vi "Actor Core.vi"(8 "error in":errorcluster, 11 "Cobra GUI in":refnum<class "Cobra GUI.lvclass">) -> (0 "error out":errorcluster={"status"=TRUE, "code"=1, "source"="Generate User Event in Panel Actor.lvlib:Panel Actor.lvclass:Actor Core.vi:5880001->GUI.lvlib:Cobra GUI.lvclass:Actor Core.vi"}, 3 "Actor out":refnum<class "Actor.lvclass">)   [LabVIEW 2019, in "Cobra GUI.lvlib" / "Cobra GUI.lvclass"]
doc: "New Cobra GUI 21.6.18"
uses:
  Cobra GUI.lvclass
  <vilib>/MGI/Panel Manager/Panel Actor/Panel Actor/Panel Actor.lvclass
  <vilib>/ActorFramework/Stop Msg/Stop Msg.lvclass
  <vilib>/MGI/Panel Manager/Panel/Panel.lvlib
  TTV Test/TTV Test/TTV Test.lvclass
  GUI 1.0/Controls/System Graphs.ctl
  GUI 1.0/GUI.lvlib
  GUI 1.0/Controls/Gauge Graphs/Compression Ratio.ctl
  GUI 1.0/Controls/Gauge Graphs/Subcooling.ctl
  GUI 1.0/Controls/Gauge Graphs/Superheat.ctl
  GUI 1.0/Controls/Gauge Graphs/Current.ctl
  GUI 1.0/Controls/Dial Gauges.ctl
  GUI Messages/Save Config Msg/Save Config Msg.lvclass
  Custom Controls/login.ctl
  <vilib>/Utility/miscctls.llb/LVPositionTypeDef.ctl
  Network Stream Messages/Open Connection Msg/Open Connection Msg.lvclass
  Network Stream/Network Stream Messages/Read Dataset Msg/Read Dataset Msg.lvclass
  Network Stream/Network Stream Messages/Close Connection Msg/Close Connection Msg.lvclass
  GUI 1.0/Controls/NS New Data.ctl
  GUI 1.0/Controls/WebDAV states.ctl
  GUI Messages/Update Msg/Update Msg.lvclass
  <vilib>/regexp/Match Regular Expression.xnode
  GUI Messages/Get IP Address Msg/Get IP Address Msg.lvclass
  <vilib>/MGI/Panel Manager/Panel/Panel/Subpanel/Subpanel.vi
  <vilib>/MGI/Panel Manager/Panel/Panel/Subpanel/Subpanel.lvclass
  C:/Program Files (x86)/National Instruments/LabVIEW 2019/vi.lib/MGI/Panel Manager/Panel Actor/Panel Actor/Panel Actor.lvclass
  C:/Program Files (x86)/National Instruments/LabVIEW 2019/vi.lib/MGI/Monitored Actor/Monitored Actor/Monitored Actor/Monitored Actor.lvclass
  C:/Program Files (x86)/National Instruments/LabVIEW 2019/vi.lib/ActorFramework/Actor/Actor.lvclass
  C:/Program Files (x86)/National Instruments/LabVIEW 2019/vi.lib/MGI/Panel Manager/Panel/Panel/Panel.lvclass
  <vilib>/ActorFramework/Actor/Actor.lvclass
  GUI 1.0/Controls/Module Key Values.ctl
  Private Controls/Module Command.ctl
  GUI 1.0/Controls/Main Waveform.ctl
  Custom Controls/Head State and Wait for the safe temp.ctl
  <vilib>/ActorFramework/Message Enqueuer/Message Enqueuer.lvclass
  <vilib>/ActorFramework/Message Priority Queue/Message Priority Queue.lvclass
  <vilib>/MGI/Panel Manager/Panel/Panel/Panel.lvclass
  <vilib>/MGI/Panel Manager/Panel/Panel Helper/Panel Helper.lvclass
  <vilib>/MGI/Panel Manager/Panel/Deferer/Deferer.lvclass
  <vilib>/MGI/Panel Manager/Panel/Panel Control Counter/Panel Control Counter.lvclass
  GUI 1.0/Controls/Module Graphs.ctl
panel:
  out "IP Address":string
  out "Connected System":string="Connected"
  out "System Info":string="Connected"
  in  "Tab Control":T1(tab)=enum."Debug"
  in  "M1 Power Drive":bool
  in  "M2 Power Drive":bool
  out "M2 Safe Temp and Head State":T2
  out "M1 Safe Temp and Head State":T2
  in  "Power On-Off":bool
  out "M2 Main Waveform":T3=[{"t0"=timestamp(3697564714.4984064 s since 1904-01-01), "dt"=1.0, "Y"=array[1697 elements]}, {"t0"=timestamp(3697564714.4984064 s since 1904-01-01), "dt"=1.0, "Y"=array[1697 elements]}, {"t0"=timestamp(3697564714.4984064 s since 1904-01-01), "dt"=1.0, "Y"=array[1697 elements]}, {"t0"=timestamp(3697564714.4984064 s since 1904-01-01), "dt"=1.0, "Y"=array[1697 elements]}]
  out "M1 Main Waveform":T3=[{"t0"=timestamp(3697564714.4984064 s since 1904-01-01), "dt"=1.0, "Y"=array[1697 elements]}, {"t0"=timestamp(3697564714.4984064 s since 1904-01-01), "dt"=1.0, "Y"=array[1697 elements]}, {"t0"=timestamp(3697564714.4984064 s since 1904-01-01), "dt"=1.0, "Y"=array[1697 elements]}, {"t0"=timestamp(3697564714.4984064 s since 1904-01-01), "dt"=1.0, "Y"=array[1697 elements]}]
  in  "M1 Commands":T4={"Set Temp"=273.15, "Read Temp"=273.15, "Package"=0, "Bin String"="", "M1 Enable"=TRUE, "TSD"=TRUE} caption="Module Commands" {"Package" items=["Ring", "Item 1", "Item 2", "Item 3"]; "Set Temp" format="%#4.1f"}
  in  "M2 Commands":T4={"Set Temp"=273.15, "Read Temp"=273.15, "Package"=0, "Bin String"="", "M1 Enable"=TRUE, "TSD"=TRUE} caption="Module Commands" {"Package" items=["Ring", "Item 1", "Item 2", "Item 3"]; "Set Temp" format="%#4.1f"}
  out "M1 Humidity":cluster{"M1 RH":dbl, "RH Threshold":dbl}(graph)={"M1 RH"=10.0, "RH Threshold"=33.76176771953824}
  out "Thermal Info":T5={"M1 Thermal State"=enum."Steady State", "M2 Thermal State"=enum."Ramp Up", "High Side RPM"=0.0, "Low Side RPM"=0.0}
  out "System Graphs":T6={"Ambient Temp"=77.534379824996, "Suction Temp"=77.78750485181808, "Condensor Temp"=77.29531729966402, "Discharge Temp"=78.09687988460064, "Bypass Steps"=72.0}
  out "Gauges":T7={"Condensing Pressure(psi)"=165.57116807812622, "Compression Ratio"=1.0119646390563775, "Subcool"=-0.3368072880168427, "Superheat"=1.4200558413526494, "Current(A)"=0.2333286882987343, "Suction Pressure(psi)"=163.4397897916897} {"Suction Pressure(psi)" scale=0.0..100.0; "Current(A)" scale=5.0..15.0 scale format="%_1f"; "Superheat" scale=0.0..100.0; "Subcool" scale=-10.0..20.0 scale format="%#4.1f"; "Compression Ratio" scale=0.0..30.0 scale format="%#.0f"; "Condensing Pressure(psi)" scale=150.0..375.0}
  in  "Graph Tab CTL":enum32{"Head #1", "Head #2"}(tab)
  out "M1 Graphs":T12={"Case Temp"=24.9375, "Evap Temp"=24.8046875, "Heater Power (%)"=0.0, "EEV Steps"=0.0, "M1 AC Load(W)"=10.492394664499656} caption="Head #1"
  out "M2 Graphs":T12 caption="Head #2"
  out "Errors":string[](array[string])=["Warning: Air not plugged in  (21 06 08 14 08)"]
  out "Event log":T13(array[cluster])=[{"Name"="Bypass Inintialized", "Time Stamp"=timestamp(3706031317.901618 s since 1904-01-01), "Code"="", "Source"="", "Value"=22160.0, "Boolean"=FALSE, "String"="Complete", "Error"=FALSE, "Warning"=FALSE, " Fault"=FALSE}, {"Name"="Timeserver not found", "Time Stamp"=timestamp(3706031309.741007 s since 1904-01-01), "Code"="", "Source"="SOM Time", "Value"=0.0, "Boolean"=FALSE, "String"="", "Error"=FALSE, "Warning"=FALSE, " Fault"=FALSE}, {"Name"="Bypass Target Change", "Time Stamp"=timestamp(3706031309.711301 s since 1904-01-01), "Code"="", "Source"="Bypass:Get Target", "Value"=110.0, "Boolean"=FALSE, "String"="", "Error"=FALSE, "Warning"=TRUE, " Fault"=FALSE}, {"Name"="Mains Frequency", "Time Stamp"=timestamp(3706031309.198055 s since 1904-01-01), "Code"="", "Source"="Init System Module", "Value"=59.9940002520096, "Boolean"=FALSE, "String"="", "Error"=FALSE, "Warning"=FALSE, " Fault"=FALSE}, {"Name"="PID Bypassed", "Time Stamp"=timestamp(3706031307.313306 s since 1904-01-01), "Code"="", "Source"="APP:Set/Send PID Bypass", "Value"=0.0, "Boolean"=FALSE, "String"="", "Error"=FALSE, "Warning"=FALSE, " Fault"=FALSE}, {"Name"="Thermal Status Change", "Time Stamp"=timestamp(3706031307.007236 s since 1904-01-01), "Code"="", "Source"="APP:Thermal Status", "Value"=0.0, "Boolean"=FALSE, "String"="", "Error"=FALSE, "Warning"=FALSE, " Fault"=FALSE}, {"Name"="Feedback Change", "Time Stamp"=timestamp(3706031306.793005 s since 1904-01-01), "Code"="", "Source"="APP:Get Feedback", "Value"=1.0, "Boolean"=FALSE, "String"="Case", "Error"=FALSE, "Warning"=FALSE, " Fault"=FALSE}, {"Name"="M1 Setpoint Change", "Time Stamp"=timestamp(3706031306.436291 s since 1904-01-01), "Code"="", "Source"="APP:Send Set Temp", "Value"=25.0, "Boolean"=FALSE, "String"="", "Error"=FALSE, "Warning"=TRUE, " Fault"=FALSE}, {"Name"="M1 Dynamic Set Point", "Time Stamp"=timestamp(3706031306.386277 s since 1904-01-01), "Code"="", "Source"="APP:Get Dynamic Set Temp", "Value"=25.0, "Boolean"=FALSE, "String"="", "Error"=FALSE, "Warning"=FALSE, " Fault"=FALSE}, {"Name"="M1 EEV Check Position", "Time Stamp"=timestamp(3706031306.325976 s since 1904-01-01), "Code"="", "Source"="", "Value"=0.0, "Boolean"=TRUE, "String"="Complete", "Error"=FALSE, "Warning"=FALSE, " Fault"=FALSE}, {"Name"="I2C TSD Freeze Timeout", "Time Stamp"=timestamp(3706031300.268274 s since 1904-01-01), "Code"="", "Source"="", "Value"=0.0, "Boolean"=FALSE, "String"="", "Error"=TRUE, "Warning"=FALSE, " Fault"=FALSE}, {"Name"="New Extra Settings Loaded", "Time Stamp"=timestamp(3706031298.435066 s since 1904-01-01), "Code"="", "Source"="", "Value"=0.0, "Boolean"=FALSE, "String"="", "Error"=FALSE, "Warning"=FALSE, " Fault"=FALSE}, {"Name"="Read Compressor Minutes", "Time Stamp"=timestamp(3706031298.210019 s since 1904-01-01), "Code"="", "Source"="", "Value"=0.0, "Boolean"=TRUE, "String"="PASS", "Error"=FALSE, "Warning"=FALSE, " Fault"=FALSE}, {"Name"="M1 EEV Check Position", "Time Stamp"=timestamp(3706031296.21211 s since 1904-01-01), "Code"="", "Source"="EEV:Check Position", "Value"=0.0, "Boolean"=FALSE, "String"="", "Error"=FALSE, "Warning"=FALSE, " Fault"=FALSE}, {"Name"="EEV PID Output", "Time Stamp"=timestamp(3706031296.161288 s since 1904-01-01), "Code"="", "Source"="APP:Send EEV PID Out", "Value"=0.0, "Boolean"=FALSE, "String"="Value Change", "Error"=FALSE, "Warning"=FALSE, " Fault"=FALSE}, {"Name"="", "Time Stamp"=timestamp(3706031296.053791 s since 1904-01-01), "Code"="", "Source"="EEV:Set Position", "Value"=0.0, "Boolean"=FALSE, "String"="", "Error"=FALSE, "Warning"=FALSE, " Fault"=FALSE}, {"Name"="", "Time Stamp"=timestamp(3706031296.000374 s since 1904-01-01), "Code"="", "Source"="EEV:Config", "Value"=0.0, "Boolean"=FALSE, "String"="", "Error"=FALSE, "Warning"=FALSE, " Fault"=FALSE}, {"Name"="M1 EEV Check Position", "Time Stamp"=timestamp(3706031294.611185 s since 1904-01-01), "Code"="", "Source"="", "Value"=2000.0, "Boolean"=TRUE, "String"="Complete", "Error"=FALSE, "Warning"=FALSE, " Fault"=FALSE}, {"Name"="M1 EEV Check Position", "Time Stamp"=timestamp(3706031294.000098 s since 1904-01-01), "Code"="", "Source"="EEV:Check Position", "Value"=0.0, "Boolean"=FALSE, "String"="", "Error"=FALSE, "Warning"=FALSE, " Fault"=FALSE}, {"Name"="EEV PID Output", "Time Stamp"=timestamp(3706031293.949764 s since 1904-01-01), "Code"="", "Source"="APP:Send EEV PID Out", "Value"=2000.0, "Boolean"=FALSE, "String"="Value Change", "Error"=FALSE, "Warning"=FALSE, " Fault"=FALSE}, {"Name"="", "Time Stamp"=timestamp(3706031293.848812 s since 1904-01-01), "Code"="", "Source"="EEV:Set Position", "Value"=0.0, "Boolean"=TRUE, "String"="", "Error"=FALSE, "Warning"=FALSE, " Fault"=FALSE}, {"Name"="EEV:Set V", "Time Stamp"=timestamp(3706031293.798386 s since 1904-01-01), "Code"="", "Source"="", "Value"=0.0, "Boolean"=FALSE, "String"="", "Error"=FALSE, "Warning"=FALSE, " Fault"=FALSE}, {"Name"="", "Time Stamp"=timestamp(3706031293.748195 s since 1904-01-01), "Code"="", "Source"="EEV:Config", "Value"=0.0, "Boolean"=FALSE, "String"="", "Error"=FALSE, "Warning"=FALSE, " Fault"=FALSE}, {"Name"="Config Loaded", "Time Stamp"=timestamp(3706031293.397414 s since 1904-01-01), "Code"="", "Source"="Config Read Initialize", "Value"=107.0, "Boolean"=FALSE, "String"="", "Error"=FALSE, "Warning"=FALSE, " Fault"=FALSE}, {"Name"="Config Read", "Time Stamp"=timestamp(3706031293.37065 s since 1904-01-01), "Code"="Found", "Source"="EEV PID", "Value"=25.0, "Boolean"=FALSE, "String"="", "Error"=FALSE, "Warning"=FALSE, " Fault"=FALSE}, {"Name"="Config Read", "Time Stamp"=timestamp(3706031293.359371 s since 1904-01-01), "Code"="Found", "Source"="Set Point Range", "Value"=-50.0, "Boolean"=FALSE, "String"="", "Error"=FALSE, "Warning"=FALSE, " Fault"=FALSE}, {"Name"="Config Value Read", "Time Stamp"=timestamp(3706031293.335439 s since 1904-01-01), "Code"="", "Source"="", "Value"=0.0, "Boolean"=TRUE, "String"="Cascade", "Error"=FALSE, "Warning"=FALSE, " Fault"=FALSE}, {"Name"="Config Value Read", "Time Stamp"=timestamp(3706031293.315639 s since 1904-01-01), "Code"="", "Source"="", "Value"=0.0, "Boolean"=TRUE, "String"="Sensors", "Error"=FALSE, "Warning"=FALSE, " Fault"=FALSE}, {"Name"="Read Saved State", "Time Stamp"=timestamp(3706031293.26891 s since 1904-01-01), "Code"="", "Source"="", "Value"=0.0, "Boolean"=FALSE, "String"="", "Error"=FALSE, "Warning"=FALSE, " Fault"=FALSE}, {"Name"="EMO Switch Detected", "Time Stamp"=timestamp(3706031293.21723 s since 1904-01-01), "Code"="", "Source"="", "Value"=0.0, "Boolean"=TRUE, "String"="", "Error"=FALSE, "Warning"=FALSE, " Fault"=FALSE}, {"Name"="Read Saved State", "Time Stamp"=timestamp(3706031293.183574 s since 1904-01-01), "Code"="", "Source"="", "Value"=0.0, "Boolean"=FALSE, "String"="", "Error"=FALSE, "Warning"=FALSE, " Fault"=FALSE}, {"Name"="FPGA Load Complete", "Time Stamp"=timestamp(3706031293.139812 s since 1904-01-01), "Code"="", "Source"="Init FPGA IO.vi", "Value"=0.0, "Boolean"=FALSE, "String"="", "Error"=FALSE, "Warning"=FALSE, " Fault"=FALSE}, {"Name"="Pressure Test", "Time Stamp"=timestamp(3706031291.136962 s since 1904-01-01), "Code"="", "Source"="Init FPGA IO 2.0.vi", "Value"=0.00022888532845044633, "Boolean"=FALSE, "String"="FAIL", "Error"=FALSE, "Warning"=TRUE, " Fault"=FALSE}, {"Name"="Stop LCD", "Time Stamp"=timestamp(3706031285.92111 s since 1904-01-01), "Code"="", "Source"="Init FPGA IO.vi", "Value"=11.0, "Boolean"=FALSE, "String"="", "Error"=FALSE, "Warning"=FALSE, " Fault"=FALSE}, {"Name"="wait", "Time Stamp"=timestamp(3706031284.919174 s since 1904-01-01), "Code"="", "Source"="Init FPGA IO.vi", "Value"=10.0, "Boolean"=FALSE, "String"="", "Error"=FALSE, "Warning"=FALSE, " Fault"=FALSE}, {"Name"="IP Address", "Time Stamp"=timestamp(3706031283.915648 s since 1904-01-01), "Code"="", "Source"="Init FPGA IO.vi", "Value"=12.0, "Boolean"=FALSE, "String"="þQ", "Error"=FALSE, "Warning"=FALSE, " Fault"=FALSE}, {"Name"="wait", "Time Stamp"=timestamp(3706031283.836404 s since 1904-01-01), "Code"="", "Source"="Init FPGA IO.vi", "Value"=10.0, "Boolean"=FALSE, "String"="", "Error"=FALSE, "Warning"=FALSE, " Fault"=FALSE}, {"Name"="Rev Display", "Time Stamp"=timestamp(3706031282.833974 s since 1904-01-01), "Code"="", "Source"="Init FPGA IO.vi", "Value"=9.0, "Boolean"=FALSE, "String"="Ver: CC 21.6.1.0", "Error"=FALSE, "Warning"=FALSE, " Fault"=FALSE}, {"Name"="wait", "Time Stamp"=timestamp(3706031282.765893 s since 1904-01-01), "Code"="", "Source"="Init FPGA IO.vi", "Value"=10.0, "Boolean"=FALSE, "String"="", "Error"=FALSE, "Warning"=FALSE, " Fault"=FALSE}, {"Name"="Chroma Display", "Time Stamp"=timestamp(3706031281.763213 s since 1904-01-01), "Code"="", "Source"="Init FPGA IO.vi", "Value"=8.0, "Boolean"=FALSE, "String"="Chroma ATE", "Error"=FALSE, "Warning"=FALSE, " Fault"=FALSE}, {"Name"="wait", "Time Stamp"=timestamp(3706031281.696552 s since 1904-01-01), "Code"="", "Source"="Init FPGA IO.vi", "Value"=10.0, "Boolean"=FALSE, "String"="", "Error"=FALSE, "Warning"=FALSE, " Fault"=FALSE}, {"Name"="Clear LCD Text", "Time Stamp"=timestamp(3706031280.693969 s since 1904-01-01), "Code"="", "Source"="Init FPGA IO.vi", "Value"=0.0, "Boolean"=FALSE, "String"="", "Error"=FALSE, "Warning"=FALSE, " Fault"=FALSE}, {"Name"="BootLoad", "Time Stamp"=timestamp(3706031279.648552 s since 1904-01-01), "Code"="", "Source"="Init FPGA IO.vi", "Value"=0.0, "Boolean"=FALSE, "String"="", "Error"=FALSE, "Warning"=FALSE, " Fault"=FALSE}, {"Name"="Extra Settings Loaded", "Time Stamp"=timestamp(3706031277.495041 s since 1904-01-01), "Code"="", "Source"="", "Value"=0.0, "Boolean"=FALSE, "String"="", "Error"=FALSE, "Warning"=FALSE, " Fault"=FALSE}, {"Name"="Warmup ", "Time Stamp"=timestamp(3706031277.461598 s since 1904-01-01), "Code"="", "Source"="Extra Settings", "Value"=0.0, "Boolean"=FALSE, "String"="", "Error"=FALSE, "Warning"=TRUE, " Fault"=FALSE}, {"Name"="Flow Curve", "Time Stamp"=timestamp(3706031277.436586 s since 1904-01-01), "Code"="", "Source"="Extra Settings", "Value"=0.0, "Boolean"=FALSE, "String"="", "Error"=FALSE, "Warning"=TRUE, " Fault"=FALSE}, {"Name"="Relative Humidity", "Time Stamp"=timestamp(3706031277.408702 s since 1904-01-01), "Code"="", "Source"="Extra Settings", "Value"=0.0, "Boolean"=TRUE, "String"="", "Error"=FALSE, "Warning"=FALSE, " Fault"=FALSE}, {"Name"="Warnings/Faults 1", "Time Stamp"=timestamp(3706031277.370367 s since 1904-01-01), "Code"="", "Source"="Extra Settings 3", "Value"=0.0, "Boolean"=TRUE, "String"="", "Error"=FALSE, "Warning"=FALSE, " Fault"=FALSE}, {"Name"="SuperHeat Settings", "Time Stamp"=timestamp(3706031277.356517 s since 1904-01-01), "Code"="", "Source"="Extra Settings 3", "Value"=0.0, "Boolean"=TRUE, "String"="", "Error"=FALSE, "Warning"=FALSE, " Fault"=FALSE}, {"Name"="Config Loaded", "Time Stamp"=timestamp(3706031277.313113 s since 1904-01-01), "Code"="", "Source"="Config Read Initialize", "Value"=74.0, "Boolean"=FALSE, "String"="", "Error"=FALSE, "Warning"=FALSE, " Fault"=FALSE}, {"Name"="Config Read", "Time Stamp"=timestamp(3706031277.287857 s since 1904-01-01), "Code"="Found", "Source"="M2 Heater PID", "Value"=0.0, "Boolean"=FALSE, "String"="", "Error"=FALSE, "Warning"=FALSE, " Fault"=FALSE}, {"Name"="Config Value Read", "Time Stamp"=timestamp(3706031277.269987 s since 1904-01-01), "Code"="", "Source"="", "Value"=0.0, "Boolean"=TRUE, "String"="Handler", "Error"=FALSE, "Warning"=FALSE, " Fault"=FALSE}] {"Value" format="%4.1f"; "Time Stamp" format="%<%x %.3X>T"}
  in  "Reboot RT":bool caption="Reboot"
  in  "Login":T14
  in  "Config Data":bool
  in  "Datalog":bool
  out "TCP Connections":T15(array[cluster])=[{"port "=1300, "remote address"="", "Connection timeout ms"=100, "Waiting for connection"=TRUE, "Waiting for Command"=FALSE, "timeout ms"=5000}, {"port "=1100, "remote address"="", "Connection timeout ms"=100, "Waiting for connection"=TRUE, "Waiting for Command"=FALSE, "timeout ms"=-1}, {"port "=1000, "remote address"="", "Connection timeout ms"=100, "Waiting for connection"=TRUE, "Waiting for Command"=FALSE, "timeout ms"=60000}, {"port "=1001, "remote address"="", "Connection timeout ms"=100, "Waiting for connection"=TRUE, "Waiting for Command"=FALSE, "timeout ms"=60000}, {"port "=2100, "remote address"="", "Connection timeout ms"=100, "Waiting for connection"=FALSE, "Waiting for Command"=FALSE, "timeout ms"=-1}, {"port "=2001, "remote address"="", "Connection timeout ms"=100, "Waiting for connection"=FALSE, "Waiting for Command"=FALSE, "timeout ms"=60000}, {"port "=2000, "remote address"="", "Connection timeout ms"=100, "Waiting for connection"=FALSE, "Waiting for Command"=FALSE, "timeout ms"=5000}]
  out "TCP commands":string[](array[string])
  in  "Cascade Compressor controls":T16 {"Manual Low Stage frequency" min=40.0 max=150.0 step=1.0; "Manual High stage frequency" min=50.0 max=150.0 step=1.0}
  in  "Manual Controls":T17
  in  "Tuning":T18={"Login TO"=10, "Fixed Y-Range"=4.0, "Average Graph"=FALSE, "Temp Unit"=FALSE, "Data Rx Timestamp"=timestamp(3700634217.978288 s since 1904-01-01), "Y-scale"=FALSE} {"Login TO" min=-1 max=1000}
  out "M2 Cluster":T19={"M2 Heater %"=0.0, "M2 Actuated"=FALSE, "M2 Error"=FALSE, "M2 Thermal Status"=enum."Steady State", "M2 Head State"=enum."Disabled", "M2 Buffer"=0.9999999999999998, "M2 Valve Output"=0.0} {"M2 Valve Output" scale=0.0..100.0; "M2 Buffer" scale=-4.0..4.0; "M2 Heater %" format="%3.0f"}
  out "M1 Cluster":T20={"M1 Heater %"=0.0, "M1 Actuated"=FALSE, "M1 Error"=FALSE, "M1 Thermal Status"=enum."Steady State", "M1 Head State"=enum."Disabled", "M1 Buffer"=0.9999999999999998, "M1 Valve Output"=0.0} {"M1 Valve Output" scale=0.0..100.0; "M1 Buffer" scale=-4.0..4.0; "M1 Heater %" format="%3.0f"}
  out "System Cluster":T21={"Serial Number"="204300076", "Compressor Hours"=59.65, "SOM Storage(MB)"=243.036, "Memory Available"=353.72, "CPU Usage"=40.953570959266244, "Software Version"="SW Version:CC 21.4.8.1", "SD card free space"=31.886, "Comp Temp"=78.09687988460064, "Sleep Timer"=-1.0, "Sleep"=TRUE, "Boot Up Time"=timestamp(3700144843.654765 s since 1904-01-01)} {"Comp Temp" format="%#.1f"; "SD card free space" format="%#4.1f"; "CPU Usage" format="%#.1f"; "Memory Available" format="%#4.1f"; "SOM Storage(MB)" format="%4.1f"; "Compressor Hours" format="%#.1f"}
  out "RT Status:":string="Running"
  out "Compressor:":string="Running"
  out "M1 State":T22={"Set Temp"=20.0, "Read Temp"=0.0, "Package"="", "Force"=0.0, "Feedback"=1} caption="M1 Status" {"Feedback" items=["Evap Temp", "Case Temp", "Intec Temp", "TSD  Temp", "Autotune", "Extra"]; "Force" format="%4.1f"; "Read Temp" format="%4.1f"; "Set Temp" format="%4.0f"}
  out "M2 State":T22={"Set Temp"=20.0, "Read Temp"=0.0, "Package"="", "Force"=0.0, "Feedback"=1} caption="M2 Status" {"Feedback" items=["Evap Temp", "Case Temp", "Intec Temp", "TSD  Temp", "Autotune", "Extra"]; "Force" format="%4.1f"; "Read Temp" format="%4.1f"; "Set Temp" format="%4.0f"}
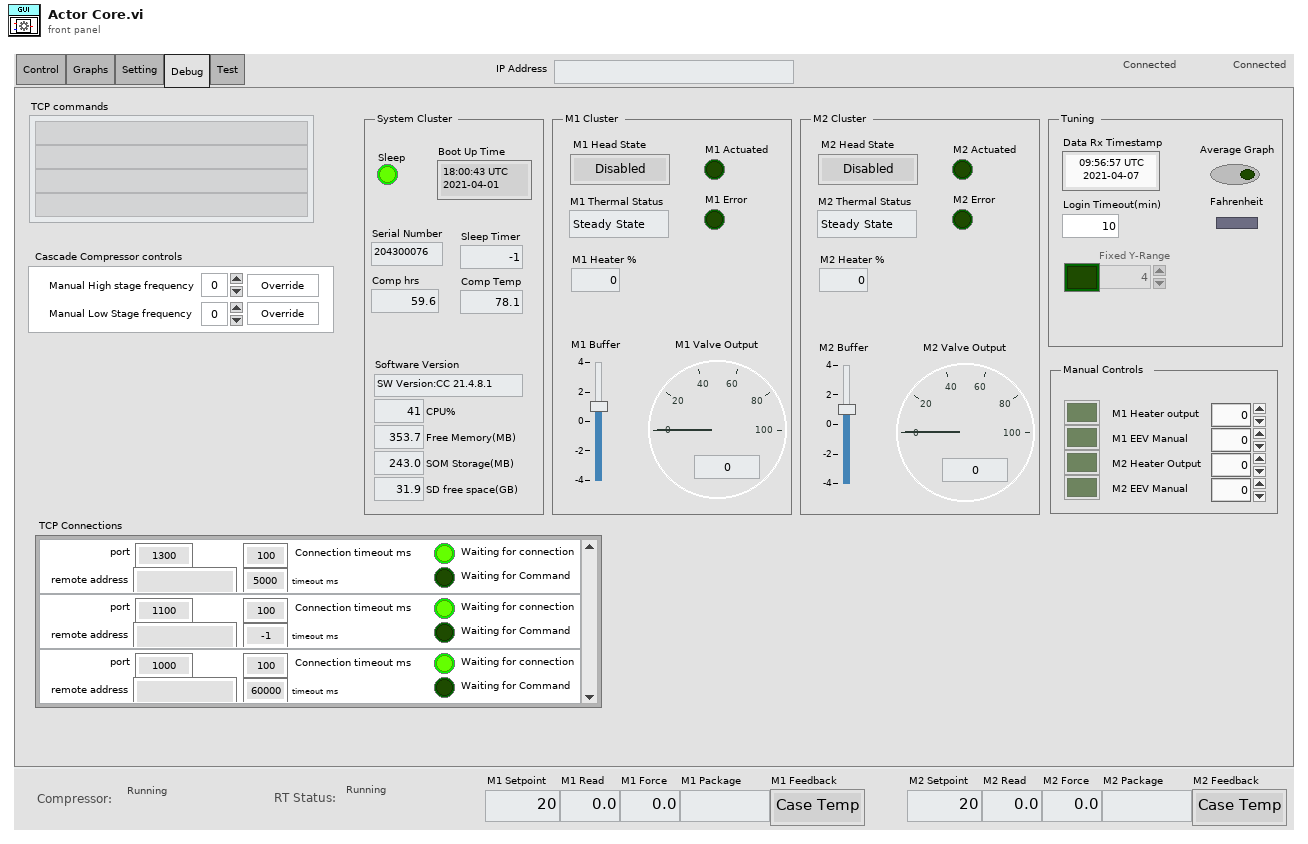
[diagram p1: front panel]
types:
  T1 = enum32{"Control", "Graphs", "Setting", "Debug", "Test"}
  T2 = typedef "GUI.lvlib/Head State and Wait for the safe temp.ctl" = bool
  T3 = typedef "GUI.lvlib/Main Waveform.ctl" = waveform(dbl)[]
  T4 = typedef "LabGUI.lvlib/Module Command.ctl" = cluster{"Set Temp":dbl[unit], "Read Temp":dbl[unit], "Package":u16, "Bin String":string, "M1 Enable":bool, "TSD":bool}
  T5 = cluster{"M1 Thermal State":enum16{"Ramp Up", "Ramp Down", "Steady State", "Ebb and Flow", "Up", "Under Load", "Cryo Mode"}, "M2 Thermal State":enum16{"Ramp Up", "Ramp Down", "Steady State", "Ebb and Flow", "Up", "Under Load", "Cryo Mode", "Shuttle Mode"}, "High Side RPM":dbl, "Low Side RPM":dbl}
  T6 = typedef "GUI.lvlib/System Graphs.ctl" = cluster{"Ambient Temp":dbl, "Suction Temp":dbl, "Condensor Temp":dbl, "Discharge Temp":dbl, "Bypass Steps":dbl}
  T7 = typedef "GUI.lvlib/Dial Gauges.ctl" = cluster{"Condensing Pressure(psi)":dbl, "Compression Ratio":T8, "Subcool":T9, "Superheat":T10, "Current(A)":T11, "Suction Pressure(psi)":dbl}
  T8 = typedef "GUI.lvlib/Compression Ratio.ctl" = dbl
  T9 = typedef "GUI.lvlib/Subcooling.ctl" = dbl
  T10 = typedef "GUI.lvlib/Superheat.ctl" = dbl
  T11 = typedef "GUI.lvlib/Current.ctl" = dbl
  T12 = typedef "GUI.lvlib/Module Graphs.ctl" = cluster{"Case Temp":dbl, "Evap Temp":dbl, "Heater Power (%)":dbl, "EEV Steps":dbl, "M1 AC Load(W)":dbl}
  T13 = cluster{"Name":string, "Time Stamp":timestamp, "Code":string, "Source":string, "Value":dbl, "Boolean":bool, "String":string, "Error":bool, "Warning":bool, " Fault":bool}[]
  T14 = typedef "GUI.lvlib/login.ctl" = bool
  T15 = cluster{"port ":u16, "remote address":string, "Connection timeout ms":i32, "Waiting for connection":bool, "Waiting for Command":bool, "timeout ms":i32}[]
  T16 = cluster{"High Stage manual speed control":bool, "Manual High stage frequency":dbl, "Low Stage manual speed control":bool, "Manual Low Stage frequency":dbl}
  T17 = cluster{"Manual Bypass Mode":bool[], "M1 Heater output":dbl, "M1 EEV Manual":u16, "M2 Heater Output":dbl, "M2 EEV Manual":u16}
  T18 = cluster{"Login TO":i32, "Fixed Y-Range":dbl, "Average Graph":bool, "Temp Unit":bool, "Data Rx Timestamp":timestamp, "Y-scale":bool}
  T19 = cluster{"M2 Heater %":dbl, "M2 Actuated":bool, "M2 Error":bool, "M2 Thermal Status":enum16{"Ramp Up", "Ramp Down", "Steady State", "Ebb and Flow", "Up", "Under Load", "Cryo Mode"}, "M2 Head State":enum16{"Disabled", "Run", "Error"}, "M2 Buffer":dbl, "M2 Valve Output":dbl}
  T20 = cluster{"M1 Heater %":dbl, "M1 Actuated":bool, "M1 Error":bool, "M1 Thermal Status":enum16{"Ramp Up", "Ramp Down", "Steady State", "Ebb and Flow", "Up", "Under Load", "Cryo Mode"}, "M1 Head State":enum16{"Disabled", "Run", "Error"}, "M1 Buffer":dbl, "M1 Valve Output":dbl}
  T21 = cluster{"Serial Number":string, "Compressor Hours":dbl, "SOM Storage(MB)":dbl, "Memory Available":dbl, "CPU Usage":dbl, "Software Version":string, "SD card free space":dbl, "Comp Temp":dbl, "Sleep Timer":dbl, "Sleep":bool, "Boot Up Time":timestamp}
  T22 = typedef "GUI.lvlib/Module Key Values.ctl" = cluster{"Set Temp":dbl, "Read Temp":dbl, "Package":string, "Force":dbl, "Feedback":u8}
  T23 = enum32{"Invalid", "Standard", "Closed", "Hidden", "Minimized", "Maximized"}
  T24 = cluster{"Event Registration Refnum":refnum<event-registration>, "Pnl Actor":refnum<event-registration>}
  T25 = enum32{"Page Enabled", "Page Disabled", "Page Disabled & Grayed"}
  T26 = typedef "LVPositionTypeDef.ctl" = cluster{"Left":i32, "Top":i32}
  T27 = typedef "GUI.lvlib/NS New Data.ctl" = enum16{"M1 Set Point", "M1 Power Drive", "M1 Feedback", "M1 Package", "M1 Enable", "M2 Set Point", "M2 Power Drive", "M2 Feedback", "M2 Package", "M2 Enable", "System Power", "Config Data", "Stop RT"}
  T28 = enum8{"Enabled", "Disabled", "Disabled and Grayed Out"}
  T29 = enum16{"Supervisor", "Engineer", "Operator", "Guest"}
  T30 = typedef "GUI.lvlib/WebDAV states.ctl" = enum16{"Open Sess", "Refresh Dir", "Create Dir", "Upload", "Download", "Delete", "Close Sess"}
  T31 = cluster{"Set Temp":dbl, "Power Drive":bool, "Feedback":u8, "Package":u16, "Enable":bool}
  T32 = typedef "GUI.lvlib/Network Data Down_set back.ctl" = cluster{"M1 Commands":cluster{"Set Temp":dbl, "Power Drive":bool, "Feedback":u8, "Package":u16, "Enable":bool}, "M2 Commands":cluster{"Set Temp":dbl, "Power Drive":bool, "Feedback":u8, "Package ":u16, "Enable":bool}, "Config Data":cluster{"Packages":cluster{"DUT Force lbf":cluster{" 0":u32, " 1":u32, " 2":u32, "3":u32, "4":u32, "5":u32, " 6":u32, "7":u32, "8":u32, "9":u32}, "DUT Names":cluster{"0":string, "1":string, "2":string, "3":string, "4":string, "5":string, "6":string, "7":string, "8":string, "9":string}}, "Heater PID":cluster{"P":dbl, "I":dbl, "D":dbl}, "Piston Settings":cluster{"Forces Slope":dbl, "Forces Intercept":dbl, "Transition Force":dbl, "Up Force":dbl, "Diameter (mm)":dbl, "Delay (ms)":dbl, "Pressure Ramp Delay (ms)":dbl}, "Safe Temps":cluster{"Minimum":i32, "Enabled":bool, "Maximum":i32}, "System Settings":cluster{"Number of Heads":i32, "60Hz Power":bool, "FTC200":bool, "AutoStartup":bool, "Purge":bool, "Sensors":bool, "HandClamp":bool, "ATE":bool, "Benchtop":bool, "Production":bool, "Refrigerant":enum16{"r404a", "r507", "r508", "r410a", "r134a"}, "Handler":bool, "Shuttle":bool, "220V":bool, "Cascade":bool, "Suction Sensor":enum16{"YCQB02H01", "YCQB02L01", "Carel"}, "Discharge Sensor":enum16{"YCQB05H01", "YCQB05L01", "Carel"}}, "Stepper Settings ":cluster{"Microstepping":enum16{"Full", "Half", "Quarter", "1/16th"}, "Velocity":u8}, "Set Point Range":cluster{"Max":dbl, "Min":dbl}, "Pedestal Check DeltaT":dbl, "Ramp Delta T":dbl, "Ramp-SS Threshold":dbl, "SS Tolerance":dbl, "EEV PID":cluster{"Ramp Up Target":dbl, "Ramp Down Target":dbl, "Steady State Target":dbl, "Output":cluster{"Max":dbl, "Min":dbl}, "EBB and Flow Temp TH":dbl, "Cryomode EEV Max":dbl, "Valve minimum opening ":dbl, "Ramp Up EEV Steps":dbl, "Ramp Down EEV Steps":dbl, "SS EEV Steps Reset":dbl, "EBB and Flow Tol":dbl, "Gains":cluster{"P":dbl, "I":dbl, "D":dbl}, "Dissabled Target":dbl, "CryoMode Gains":cluster{"P":dbl, "I":dbl, "D":dbl}, "M1 SuperHeat Setpoint":dbl, "M2 Gains":cluster{"P":dbl, "I":dbl, "D":dbl}, "Flow Curve":enum16{""}}, "Sleep Timeout":dbl, "Bypass Values":cluster{"Bypass Valve":bool, "Flow Curve":enum16{"0", "1"}, "Output":cluster{"Max":u32, "Min":u32}, "Feedback":enum16{"Temperature", "Pressure", "Superheat", "Pressure 2.0"}, "Cyth Bypass":bool, "PID":cluster{"P":dbl, "I":dbl, "D":dbl}, "Pressure setpoint":i16, "Cryo Temp":i16, "Superheat Setpoint":i16, "Cryo Setpoint":i16}, "Default Temp":dbl, "InTEC":cluster{"Enabled":bool, "IP":string, "Port":u16}, "M1 TSD":cluster{"Gain":dbl, "Offset":dbl, "V Offset ":dbl}, "M2 TSD":cluster{"Gain":dbl, "Offset":dbl, "V Offset ":dbl}, "M1 T-Case Calibration":cluster{"Gain":dbl, "Offset":dbl}, "M2 T-Case Calibration":cluster{"Gain":dbl, "Offset":dbl}, "Heater PID TSD":cluster{"P":dbl, "I":dbl, "D":dbl}, "M2 Heater PID":cluster{"P":dbl, "I":dbl, "D":dbl}}, "System Power On Off":bool, "New Data":T27, "Stop RT":bool}
  T33 = typedef "GUI.lvlib/System Status.ctl" = cluster{"Power On Off":bool, "Discharge Temp":dbl, "Liquid Temp":dbl, "Suction Temp":dbl, "Ambient Temp":dbl, "Sleep":bool, "System Status":u16, "M1 Actuated":bool, "M2 Actuated":bool, "Sleep Timer":dbl, "M1 Bin":cluster{"Bin String":string, "Bin Color":u16}, "M2 Bin":cluster{"Bin String":string, "Bin Color":u16}, "Discharge Pressure":dbl, "Suction Pressure":dbl, "Compression Ratio":dbl, "Compressor Amps":dbl, "Compressor Hours":dbl, "Bypass Steps":u16, "SubCooling":dbl, "SuperHeat":dbl, "Serial Number":string, "EMO detected":bool, "EMO Tripped":bool, "Thermal cutoff":bool, "Thermal cutoff 2":bool, "High Pressure switch":bool, "Running Time":timestamp, "SOM Status":cluster{"Boot Up Time":timestamp, "Software Version":string, "CPU Usage":dbl, "Memory Available":dbl, "SD card free space":dbl, "SOM Storage":dbl}, "Cascade Extra":cluster{"Discharge Temp High Side":dbl, "Suction Temp High Side":dbl, "Liquid Temp High side":dbl, "Discharge Pressure 2":dbl, "Suction Pressure 2":dbl, "Low Side RPM":dbl, "High Side RPM":dbl}}
  T34 = typedef "GUI.lvlib/Module Status.ctl" = cluster{"Case Temp":dbl, "Evap Temp":dbl, "Heater %":dbl, "EEV Steps":u32, "Set Temp":dbl, "Feedback":u8, "Power Drive":bool, "Piston Volts":dbl, "Safe Temp":bool, "Power":bool, "Thermal State":u16, "Error":bool, "In tollerance":bool, "Head State":u16, "Piston Force":dbl, "Package":string, "Dynamic SV":dbl, "PV":dbl, "TSD Temp":dbl, "DC Load Watts":dbl, "AC Load Watts":dbl, "Intec Feedback":dbl}
  T35 = typedef "NI_WebDAV.lvlib/FileInfo.ctl" = cluster{"type":string, "size":u64, "last modification":timestamp, "display name":string, "uri":string}
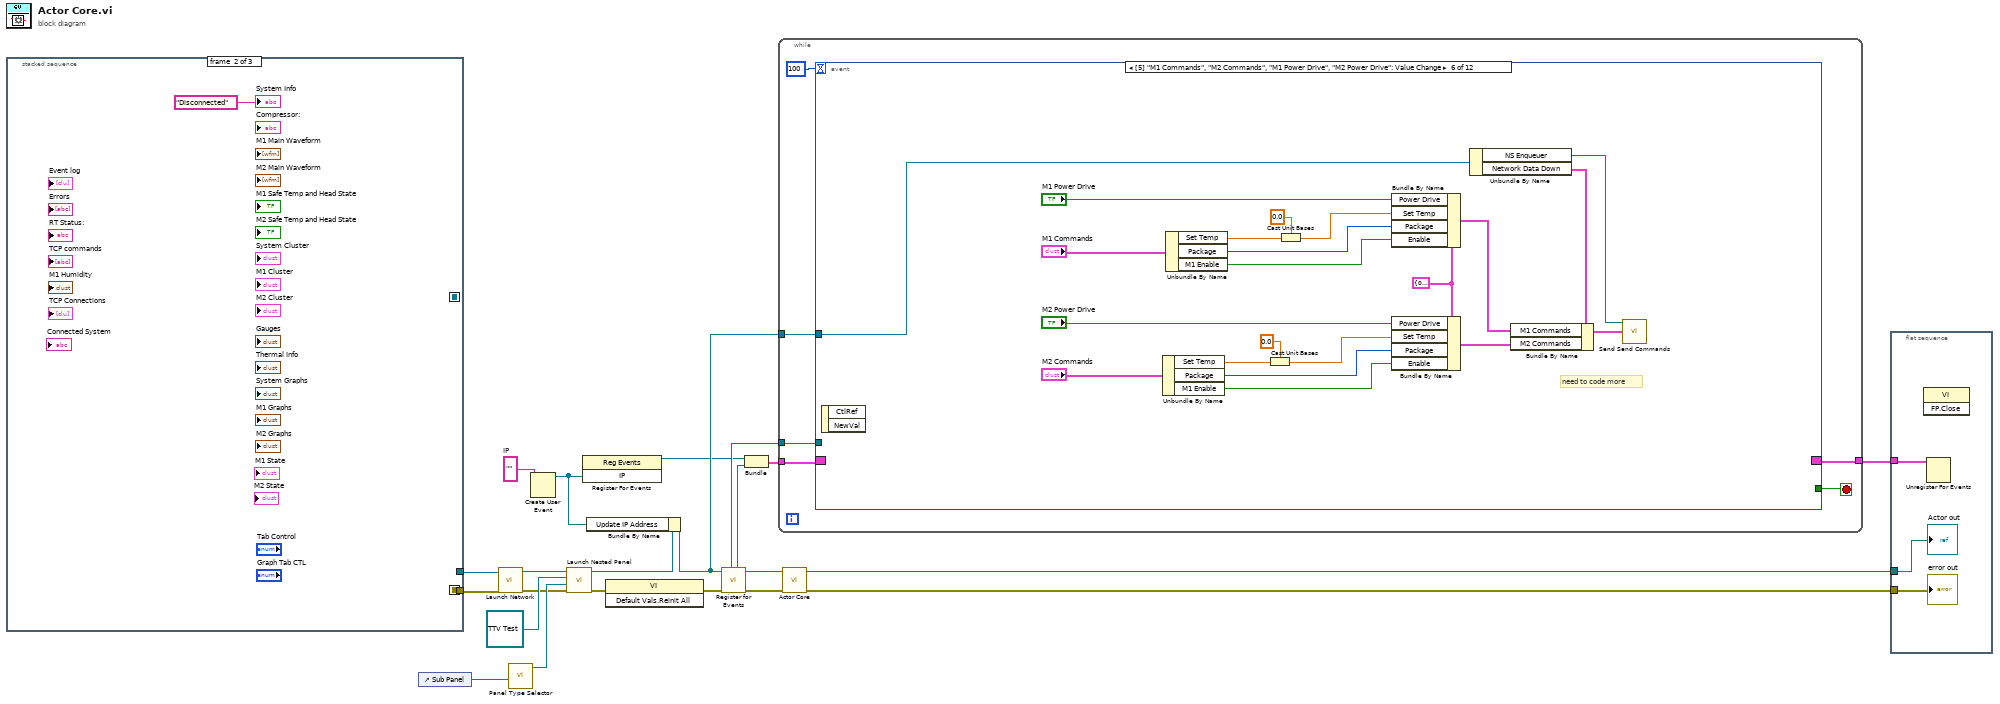
[diagram p0: block diagram]
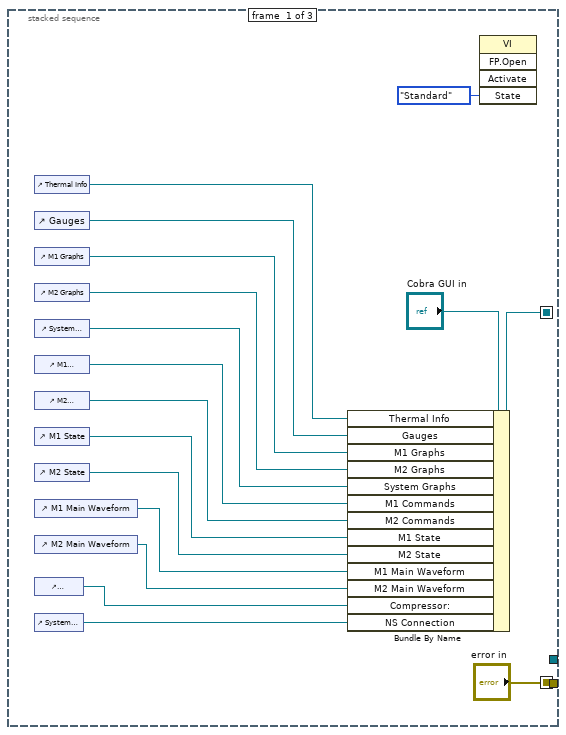
[diagram p2: hidden frame]
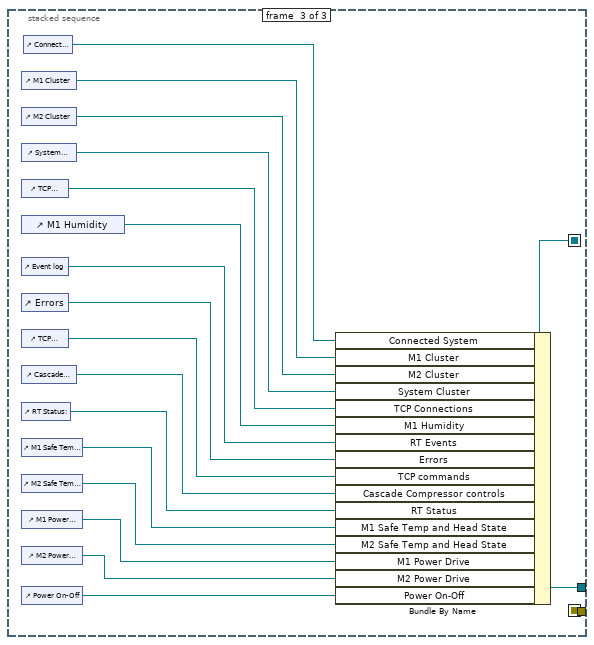
[diagram p3: hidden frame]
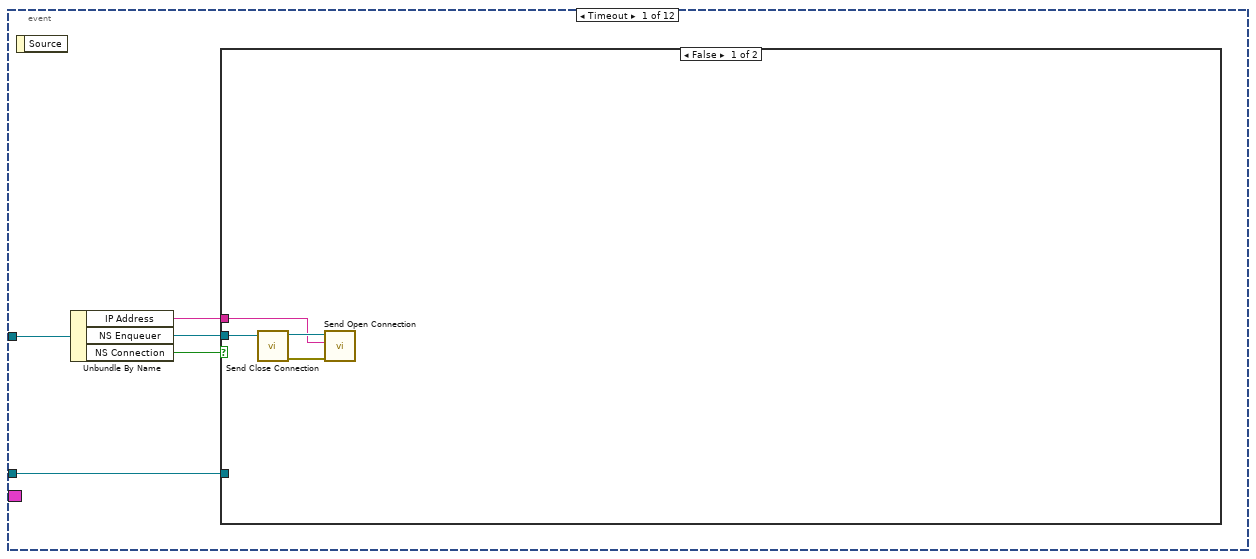
[diagram p4: hidden frame]
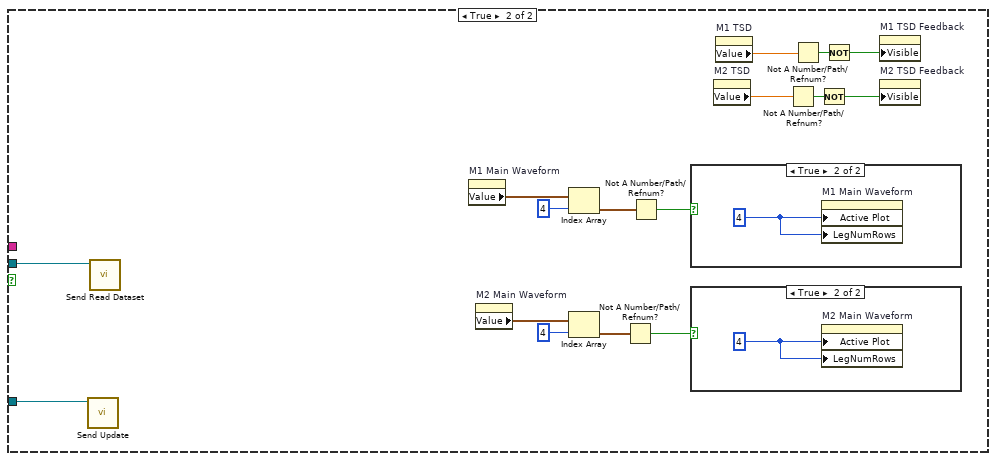
[diagram p5: hidden frame]
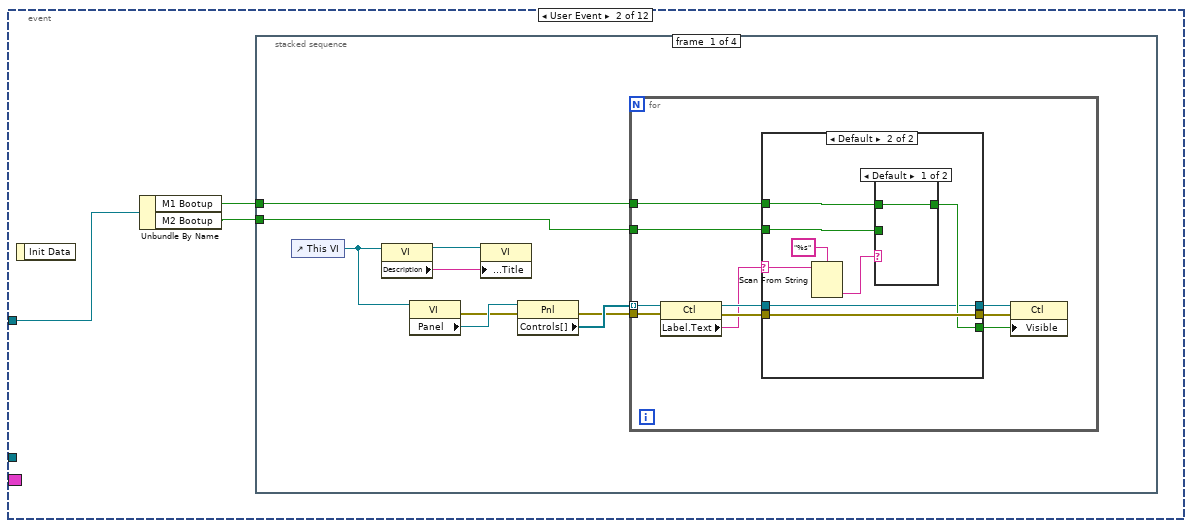
[diagram p8: hidden frame]
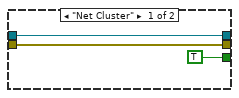
[diagram p9: hidden frame]
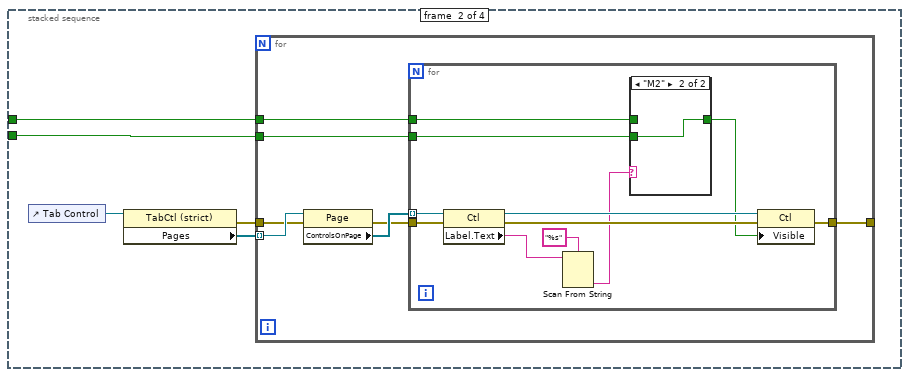
[diagram p11: hidden frame]
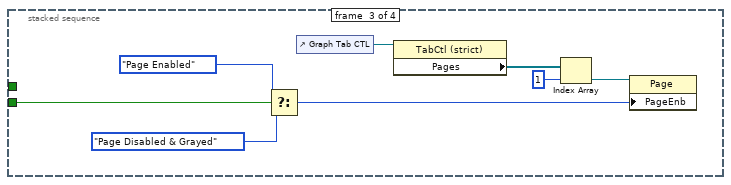
[diagram p13: hidden frame]
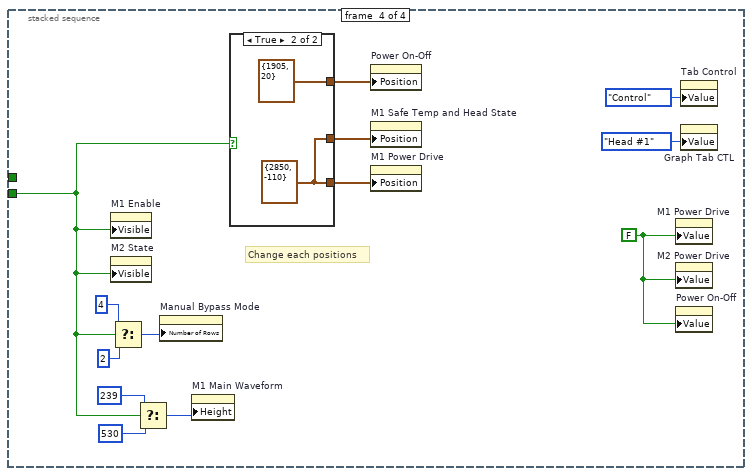
[diagram p14: hidden frame]
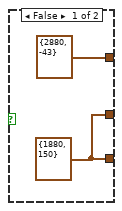
[diagram p15: hidden frame]
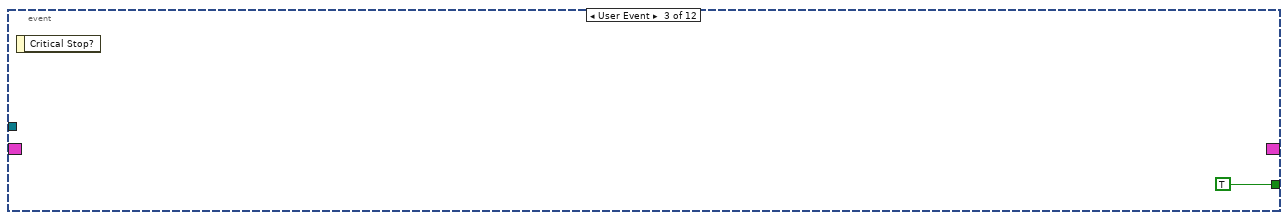
[diagram p16: hidden frame]
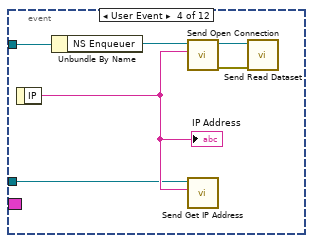
[diagram p17: hidden frame]
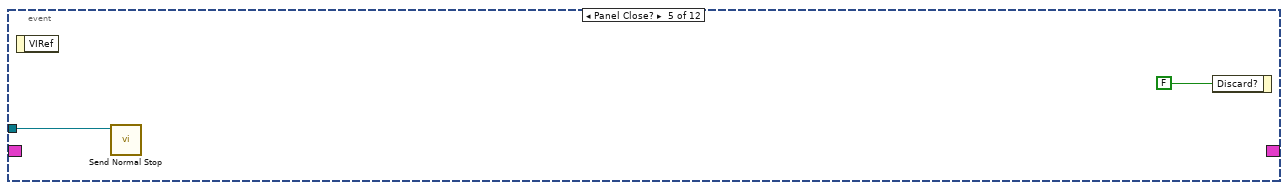
[diagram p18: hidden frame]
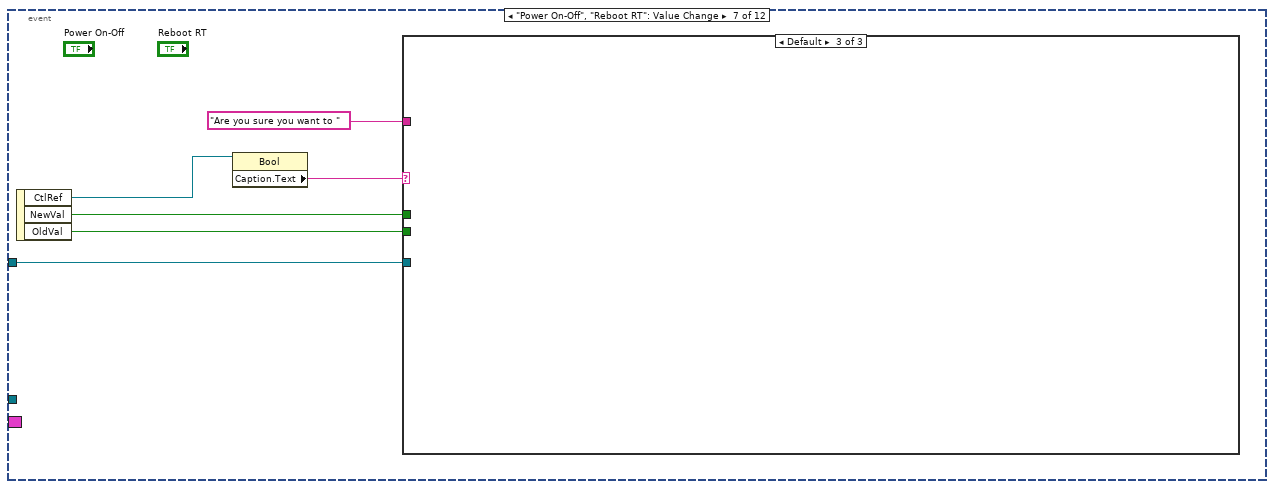
[diagram p19: hidden frame]
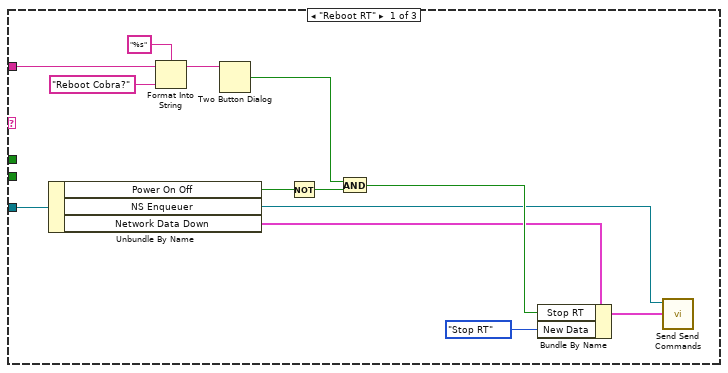
[diagram p20: hidden frame]
diagram:
  w9 = ""  # IP
  n1 = stacked-sequence {
    seq-local: ["error in" _ _] -> [_ _ w57]
    seq-local: [w36 _ _] -> [_ _ w58]
    tunnel: [_ _ w57] -> w2
    tunnel: [_ _ w59] -> w1
    frame #0 {
      n2 = control-ref of="Thermal Info"() -> (w25:refnum<vi>)
      n3 = control-ref of="Gauges"() -> (w24:refnum<vi>)
      n4 = control-ref of="M1 Graphs"() -> (w26:refnum<vi>)
      n5 = control-ref of="M2 Graphs"() -> (w27:refnum<vi>)
      n6 = control-ref of="System Graphs"() -> (w28:refnum<vi>)
      n7 = control-ref of="M1 Commands"() -> (w30:refnum<vi>)
      n8 = control-ref of="M2 Commands"() -> (w31:refnum<vi>)
      n9 = control-ref of="M1 State"() -> (w32:refnum<vi>)
      n10 = control-ref of="M2 State"() -> (w33:refnum<vi>)
      n11 = control-ref of="M1 Main Waveform"() -> (w34:refnum<vi>)
      n12 = control-ref of="M2 Main Waveform"() -> (w35:refnum<vi>)
      n13 = control-ref of="Compressor:"() -> (w37:refnum<vi>)
      n14 = control-ref of="System Info"() -> (w38:refnum<vi>)
      n15 = Bundle By Name(cluster="Cobra GUI in", "Thermal Info"=w25, "Gauges"=w24, "M1 Graphs"=w26, "M2 Graphs"=w27, "System Graphs"=w28, "M1 Commands"=w30, "M2 Commands"=w31, "M1 State"=w32, "M2 State"=w33, "M1 Main Waveform"=w34, "M2 Main Waveform"=w35, "Compressor:"=w37, "NS Connection"=w38) -> (w36:refnum<class "Cobra GUI.lvclass">)
      n16 = invoke class="VI" method="FP.Open"("State"=T23."Standard") -> ()  [unwired: 4 in, 5 out]
    }
    frame #1 {
      "System Info" <- "Disconnected" ("System Info")
    }
    frame #2 {
      n17 = control-ref of="M1 Cluster"() -> (w49:refnum<vi>)
      n18 = control-ref of="M2 Cluster"() -> (w50:refnum<vi>)
      n19 = control-ref of="System Cluster"() -> (w51:refnum<vi>)
      n20 = control-ref of="TCP Connections"() -> (w42:refnum<vi>)
      n21 = control-ref of="M1 Humidity"() -> (w43:refnum<vi>)
      n22 = control-ref of="Event log"() -> (w46:refnum<vi>)
      n23 = control-ref of="Errors"() -> (w47:refnum<vi>)
      n24 = control-ref of="TCP commands"() -> (w44:refnum<vi>)
      n25 = control-ref of="Cascade Compressor controls"() -> (w52:refnum<vi>)
      n26 = control-ref of="RT Status:"() -> (w45:refnum<vi>)
      n27 = control-ref of="M1 Safe Temp and Head State"() -> (w53:refnum<vi>)
      n28 = control-ref of="M2 Safe Temp and Head State"() -> (w54:refnum<vi>)
      n29 = control-ref of="M1 Power Drive"() -> (w55:refnum<vi>)
      n30 = control-ref of="M2 Power Drive"() -> (w56:refnum<vi>)
      n31 = control-ref of="Power On-Off"() -> (w48:refnum<vi>)
      n32 = control-ref of="Connected System"() -> (w41:refnum<vi>)
      n33 = Bundle By Name(cluster=w58, "Connected System"=w41, "M1 Cluster"=w49, "M2 Cluster"=w50, "System Cluster"=w51, "TCP Connections"=w42, "M1 Humidity"=w43, "RT Events"=w46, "Errors"=w47, "TCP commands"=w44, "Cascade Compressor controls"=w52, "RT Status"=w45, "M1 Safe Temp and Head State"=w53, "M2 Safe Temp and Head State"=w54, "M1 Power Drive"=w55, "M2 Power Drive"=w56, "Power On-Off"=w48) -> (w59:refnum<class "Cobra GUI.lvclass">)
    }
  }
  n34 = control-ref of="Sub Panel"() -> (w18:refnum<vi>)
  n35 = call-dynamic "Launch Network.vi"("error in (no error)"=w2, "Cobra GUI in"=w1) -> ("error out"=w13:errorcluster, "Cobra GUI out"=w12:refnum<class "Cobra GUI.lvclass">)  [unwired: 8 in]
  n36 = call-poly <vilib>:"Panel Type Selector.vi"("Sub Panel"=w18) -> ("Subpanel Out"=w19:refnum<class "Subpanel.lvclass">)  [unwired: 9 in, 1 out]
  n37 = Create User Event(user event datatype=w9) -> (user event=w7:refnum<user-event>)  [unwired: 1 in, 1 out]
  n38 = call <vilib>:"Launch Nested Panel.vi"("error in (no error)"=w13, "Panel"=w19, "Nested Panel Actor"=refnum<class "TTV Test.lvclass"> refnum ("TTV Test.lvlib:TTV Test.lvclass"), "Panel Actor in"=w12) -> ("error out"=w11:errorcluster, "Panel Actor out"=w8:refnum<class "Cobra GUI.lvclass">)  [unwired: 4 in, 2 out]
  n39 = register-events(w7) -> (reference out=w5:refnum<event-registration>)  [unwired: 2 in, 1 out]
  n40 = Bundle By Name(cluster=w8, "Update IP Address"=w7) -> (w6:refnum<class "Cobra GUI.lvclass">)
  n41 = invoke class="VI" method="Default Vals.Reinit All"(error in=w11) -> (error out=w10:errorcluster)  [unwired: 2 in, 2 out]
  n42 = call <vilib>:"Register for Events.vi"("Error In"=w10, "Panel Actor in"=w6) -> ("Error Out"=w22:errorcluster, "Panel Actor out"=w16:refnum<class "Cobra GUI.lvclass">, "Pnl Actor"=w4:refnum<event-registration>, "Self Enqueuer"=w21:refnum<class "Message Enqueuer.lvclass">)  [unwired: 6 in]
  n43 = Bundle("Event Registration Refnum"=w5, "Pnl Actor"=w4) -> (w3:T24)  [unwired: 1 in]
  n44 = while {
    tunnel: w21 -> [w63]
    tunnel: [w64] -> w20
    tunnel: w6 -> [w62]
    tunnel: w3 -> [w60]
    stop <- w65 stop-if-true
    n45 = event shown="[5] \"M1 Commands\", \"M2 Commands\", \"M1 Power Drive\", \"M2 Power Drive\": Value Change" {
      selector: w60 -> [_ _ _ _ _ _ _ _ _ _ _ _]
      dyn-events: [_ _ _ _ _ _ _ _ _ _ _ _] -> w64
      timeout: 100 -> [_ _ _ _ _ _ _ _ _ _ _ _]
      tunnel: [_ _ TRUE _ _ _ _ _ _ _ _ _] -> w65
      tunnel: w63 -> [w69 _ _ w182 w186 _ _ w256 _ _ _ _]
      tunnel: w62 -> [w70 w93 _ w179 _ w191 w208 _ w260 w359 _ w503]
      event Timeout {
        n46 = event-data() -> ()  [unwired: 1 in, 1 out]
        n47 = Unbundle By Name(w70) -> ("IP Address"=w66:string, "NS Enqueuer"=w68:refnum<class "Message Enqueuer.lvclass">, "NS Connection"=w67:bool)
        n48 = case shown="False" w67 {
          tunnel: w68 -> [w74 w90]
          tunnel: w66 -> [w71 _]
          tunnel: w69 -> [_ w89]
          frame False {
            n49 = call "Send Close Connection.vi"("Message Enqueuer"=w74) -> ("error out"=w72:errorcluster, "Message Enqueuer out"=w73:refnum<class "Message Enqueuer.lvclass">)  [unwired: 9 in]
            n50 = call "Send Open Connection.vi"("error in (no error)"=w72, "IP"=w71, "Message Enqueuer"=w73) -> ()  [unwired: 7 in, 2 out]
          }
          frame True {
            n51 = call "Send Update.vi"("Message Enqueuer"=w89) -> ()  [unwired: 9 in, 2 out]
            n52 = call "Send Read Dataset.vi"("Message Enqueuer"=w90) -> ()  [unwired: 9 in, 2 out]
            n53 = property on="M1 Main Waveform" class="WFChart (strict)"() -> ("Value"=w83:T3)  [unwired: 2 in, 2 out]
            n54 = property on="M2 Main Waveform" class="WFChart (strict)"() -> ("Value"=w79:T3)  [unwired: 2 in, 2 out]
            n55 = Index Array(array=w83, index=4) -> (element=w82:waveform(dbl))
            n56 = Index Array(array=w79, index=4) -> (element=w80:waveform(dbl))
            n57 = Not A Number/Path/Refnum?(number/path/refnum=w80) -> (NaN/Path/Refnum?=w78:bool)
            n58 = Not A Number/Path/Refnum?(number/path/refnum=w82) -> (NaN/Path/Refnum?=w81:bool)
            n59 = case shown="True" w81 {
              frame False {
              }
              frame True {
                w92 = u32 4 ("Active Plot")
                n60 = property on="M1 Main Waveform" class="WFChart (strict)"("Active Plot"=w92, "LegNumRows"=w92) -> ()  [unwired: 2 in, 2 out]
              }
            }
            n61 = case shown="True" w78 {
              frame False {
              }
              frame True {
                w91 = u32 4 ("Active Plot")
                n62 = property on="M2 Main Waveform" class="WFChart (strict)"("Active Plot"=w91, "LegNumRows"=w91) -> ()  [unwired: 2 in, 2 out]
              }
            }
            n63 = property on="M2 TSD" class="DigNum (strict)"() -> ("Value"=w87:dbl)  [unwired: 2 in, 2 out]
            n64 = property on="M1 TSD" class="DigNum (strict)"() -> ("Value"=w85:dbl)  [unwired: 2 in, 2 out]
            n65 = Not A Number/Path/Refnum?(number/path/refnum=w87) -> (NaN/Path/Refnum?=w75:bool)
            n66 = Not A Number/Path/Refnum?(number/path/refnum=w85) -> (NaN/Path/Refnum?=w86:bool)
            n67 = Not(x=w75) -> (.not. x?=w88:bool)
            n68 = Not(x=w86) -> (.not. x?=w84:bool)
            n69 = property on="M1 TSD Feedback" class="Bool (strict)"("Visible"=w84) -> ()  [unwired: 2 in, 2 out]
            n70 = property on="M2 TSD Feedback" class="Bool (strict)"("Visible"=w88) -> ()  [unwired: 2 in, 2 out]
          }
        }
      }
      event User Event {
        n71 = event-data() -> ()  [unwired: 1 in, 1 out]
        n72 = Unbundle By Name(w93) -> ("M1 Bootup"=w94:bool, "M2 Bootup"=w95:bool)
        n73 = stacked-sequence {
          tunnel: w95 -> [w96 w129 w153 w162]
          tunnel: w94 -> [w97 w128 _ _]
          frame #0 {
            n74 = control-ref of="This VI"() -> (w99:refnum<vi>)
            n75 = property class="VI"(reference=w99) -> (reference out=w103:refnum<vi>, "Description"=w104:string)  [unwired: 1 in, 1 out]
            n76 = property class="VI"(reference=w99) -> (error out=w100:errorcluster, "Panel"=w102:refnum<vi>)  [unwired: 1 in, 1 out]
            n77 = property class="VI"(reference=w103, "Front Panel.Title"=w104) -> ()  [unwired: 1 in, 2 out]
            n78 = property class="Pnl"(reference=w102, error in=w100) -> (error out=w98:errorcluster, "Controls[]"=w101:refnum<vi>[])  [unwired: 1 out]
            n79 = for {
              tunnel: w101 -> [w114] mode=indexing
              tunnel: w97 -> [w111]
              tunnel: w96 -> [w110]
              tunnel: w98 -> [w105]
              n80 = property class="Ctl"(reference=w114, error in=w105) -> (reference out=w112:refnum<vi>, error out=w113:errorcluster, "Label.Text"=w109:string)
              n81 = case shown="Default" w109 {
                selector: w109 -> [_ w120]
                tunnel: [w115 w123] -> w108
                tunnel: w113 -> [w115 w123]
                tunnel: w112 -> [w116 w118]
                tunnel: w111 -> [_ w122]
                tunnel: w110 -> [_ w121]
                tunnel: [TRUE ("Network Connection") w119] -> w107
                tunnel: [w116 w118] -> w106
                frame "Net Cluster" {
                }
                frame Default {
                  n82 = Scan From String(format string="%s", input string=w120) -> (output 1=w125:string)  [unwired: 3 in, 3 out]
                  n83 = case shown="Default" w125 {
                    tunnel: [w126 w127] -> w119
                    tunnel: w122 -> [w126 _]
                    tunnel: w121 -> [_ w127]
                    frame Default {
                    }
                    frame "M2" {
                    }
                  }
                }
              }
              n84 = property class="Ctl"(reference=w106, error in=w108, "Visible"=w107) -> ()  [unwired: 2 out]
            }
          }
          frame #1 {
            n85 = control-ref of="Tab Control"() -> (w130:refnum<vi>)
            n86 = property class="TabCtl (strict)"(reference=w130) -> (error out=w132:errorcluster, "Pages"=w131:refnum<vi>[])  [unwired: 1 in, 1 out]
            n87 = for {
              tunnel: w131 -> [w139] mode=indexing
              tunnel: w132 -> [w137]
              tunnel: w129 -> [w135]
              tunnel: w128 -> [w134]
              tunnel: [w133] -> _
              n88 = property class="Page"(reference=w139, error in=w137) -> (error out=w136:errorcluster, "ControlsOnPage"=w138:refnum<vi>[])  [unwired: 1 out]
              n89 = for {
                tunnel: w138 -> [w150] mode=indexing
                tunnel: w136 -> [w149]
                tunnel: w135 -> [w148]
                tunnel: w134 -> [w147]
                tunnel: [w146] -> w133
                n90 = property class="Ctl"(reference=w150, error in=w149) -> (reference out=w144:refnum<vi>, error out=w143:errorcluster, "Label.Text"=w141:string)
                n91 = Scan From String(format string="%s", input string=w141) -> (output 1=w142:string)  [unwired: 3 in, 3 out]
                n92 = case shown="\"M2\"" w142 {
                  tunnel: w147 -> [w151 _]
                  tunnel: w148 -> [_ w152]
                  tunnel: [w151 w152] -> w140
                  frame Default {
                  }
                  frame "M2" {
                  }
                }
                n93 = property class="Ctl"(reference=w144, error in=w143, "Visible"=w140) -> (error out=w146:errorcluster)  [unwired: 1 out]
              }
            }
          }
          frame #2 {
            n94 = Select(t=T25."Page Enabled" ("Page Enabled State"), s=w153, f=T25."Page Disabled & Grayed" ("Page Enabled State")) -> (s? t:f=w157:T25)
            n95 = control-ref of="Graph Tab CTL"() -> (w160:refnum<vi>)
            n96 = property class="TabCtl (strict)"(reference=w160) -> ("Pages"=w158:refnum<vi>[])  [unwired: 1 in, 2 out]
            n97 = Index Array(array=w158, index=1) -> (element=w159:refnum<vi>)
            n98 = property class="Page"(reference=w159, "PageEnb"=w157) -> ()  [unwired: 1 in, 2 out]
          }
          frame #3 {
            w161 = FALSE ("M1 Power Drive")
            # "Change each positions"
            n99 = property on="M1 Enable" class="Bool (strict)"("Visible"=w162) -> ()  [unwired: 2 in, 2 out]
            n100 = property on="M2 State" class="Clust (strict)"("Visible"=w162) -> ()  [unwired: 2 in, 2 out]
            n101 = Select(t=u32 4 ("Number of Rows"), s=w162, f=u32 2 ("Number of Rows")) -> (s? t:f=w171:u32)
            n102 = Select(t=u32 239 ("Plot Area:Size:Height"), s=w162, f=u32 530 ("Plot Area:Size:Height")) -> (s? t:f=w168:u32)
            n103 = property on="Manual Bypass Mode" class="Arr (strict)"("Number of Rows"=w171) -> ()  [unwired: 2 in, 2 out]
            n104 = property on="M1 Main Waveform" class="WFChart (strict)"("Height"=w168) -> ()  [unwired: 2 in, 2 out]
            n105 = case shown="True" w162 {
              tunnel: [w175 w177] -> w163
              tunnel: [w175 w177] -> w164
              tunnel: [T26 {"Left"=2880, "Top"=-43} ("Position") T26 {"Left"=1905, "Top"=20} ("Position")] -> w165
              frame False {
                w175 = T26 {"Left"=1880, "Top"=150} ("Position")
              }
              frame True {
                w177 = T26 {"Left"=2850, "Top"=-110} ("Position")
              }
            }
            n106 = property on="Power On-Off" class="Bool (strict)"("Position"=w165) -> ()  [unwired: 2 in, 2 out]
            n107 = property on="M1 Safe Temp and Head State" class="Bool (strict)"("Position"=w164) -> ()  [unwired: 2 in, 2 out]
            n108 = property on="M1 Power Drive" class="Bool (strict)"("Position"=w163) -> ()  [unwired: 2 in, 2 out]
            n109 = property on="M1 Power Drive" class="Bool (strict)"("Value"=w161) -> ()  [unwired: 2 in, 2 out]
            n110 = property on="M2 Power Drive" class="Bool (strict)"("Value"=w161) -> ()  [unwired: 2 in, 2 out]
            n111 = property on="Power On-Off" class="Bool (strict)"("Value"=w161) -> ()  [unwired: 2 in, 2 out]
            n112 = property on="Tab Control" class="TabCtl (strict)"("Value"=T1."Control" ("Tab Control")) -> ()  [unwired: 2 in, 2 out]
            n113 = property on="Graph Tab CTL" class="TabCtl (strict)"("Value"=enum32{"Head #1", "Head #2"}."Head #1" ("Graph Tab CTL")) -> ()  [unwired: 2 in, 2 out]
          }
        }
      }
      event User Event {
        n114 = event-data() -> ()  [unwired: 1 in, 1 out]
      }
      event User Event {
        n115 = event-data() -> ("IP"=w183:string)  [unwired: 1 in]
        "IP Address" <- w183
        n116 = Unbundle By Name(w179) -> ("NS Enqueuer"=w184:refnum<class "Message Enqueuer.lvclass">)
        n117 = call "Send Open Connection.vi"("IP"=w183, "Message Enqueuer"=w184) -> ("error out"=w181:errorcluster, "Message Enqueuer out"=w180:refnum<class "Message Enqueuer.lvclass">)  [unwired: 8 in]
        n118 = call "Send Get IP Address.vi"("IP Address"=w183, "Message Enqueuer"=w182) -> ()  [unwired: 8 in, 2 out]
        n119 = call "Send Read Dataset.vi"("error in (no error)"=w181, "Message Enqueuer"=w180) -> ()  [unwired: 8 in, 2 out]
      }
      event Panel Close? {
        n120 = event-data() -> ()  [unwired: 1 in, 1 out]
        n121 = call <vilib>:"Send Normal Stop.vi"("Message Enqueuer"=w186) -> ()  [unwired: 10 in, 1 out]
        n122 = event-data("Discard?"=FALSE) -> ()  [unwired: 1 in, 1 out]
      }
      event "M1 Power Drive", "M2 Power Drive": Value Change {
        w207 = T31 {"Set Temp"=0.0, "Power Drive"=FALSE, "Feedback"=0, "Package"=0, "Enable"=FALSE} ("M1 Write Commands")
        # "need to code more"
        n123 = event-data() -> ()  [unwired: 1 in, 2 out]
        n124 = Unbundle By Name("M2 Commands") -> ("Set Temp"=w196:dbl[unit], "Package"=w194:u16, "M1 Enable"=w193:bool)
        n125 = Unbundle By Name("M1 Commands") -> ("Set Temp"=w203:dbl[unit], "Package"=w201:u16, "M1 Enable"=w200:bool)
        n126 = Cast Unit Bases(0:w196, 1:0.0 ("Set Temp")) -> (2:w195:dbl)
        n127 = Cast Unit Bases(0:w203, 1:0.0 ("Set Temp")) -> (2:w202:dbl)
        n128 = Bundle By Name(cluster=w207, "Power Drive"="M1 Power Drive", "Set Temp"=w202, "Package"=w201, "Enable"=w200) -> (w189:T31)
        n129 = Bundle By Name(cluster=w207, "Power Drive"="M2 Power Drive", "Set Temp"=w195, "Package"=w194, "Enable"=w193) -> (w188:T31)
        n130 = Unbundle By Name(w191) -> ("NS Enqueuer"=w190:refnum<class "Message Enqueuer.lvclass">, "Network Data Down"=w187:T32)
        n131 = Bundle By Name(cluster=w187, "M1 Commands"=w189, "M2 Commands"=w188) -> (w192:T32)
        n132 = call "Send Send Commands.vi"("Set Temp"=w192, "Message Enqueuer"=w190) -> ()  [unwired: 8 in, 2 out]
      }
      event "Power On-Off", "Reboot RT": Value Change {
        n133 = event-data() -> ("CtlRef"=w213:refnum<vi>, "NewVal"=w210:bool, "OldVal"=w209:bool)  [unwired: 1 in]
        n134 = property class="Bool"(reference=w213) -> ("Caption.Text"=w212:string)  [unwired: 1 in, 2 out]
        n135 = case shown="Default" w212 {
          tunnel: "Are you sure you want to " ("message") -> [w223 w236 _]
          tunnel: w209 -> [_ w235 _]
          tunnel: w208 -> [w220 w228 _]
          tunnel: w210 -> [_ w233 _]
          frame "Reboot RT" {
            n136 = Unbundle By Name(w220) -> ("Power On Off"=w226:bool, "NS Enqueuer"=w215:refnum<class "Message Enqueuer.lvclass">, "Network Data Down"=w214:T32)
            n137 = Format Into String(format string="%s", initial string=w223, "Reboot Cobra?" ("message")) -> (resulting string=w222:string)  [unwired: 1 in, 1 out]
            n138 = Two Button Dialog(message=w222) -> (T button?=w216:bool)  [unwired: 2 in]
            n139 = Not(x=w226) -> (.not. x?=w217:bool)
            n140 = And(x=w216, y=w217) -> (x .and. y?=w219:bool)
            n141 = Bundle By Name(cluster=w214, "Stop RT"=w219, "New Data"=NS_New_Data."Stop RT") -> (w221:T32)
            n142 = call "Send Send Commands.vi"("Set Temp"=w221, "Message Enqueuer"=w215) -> ()  [unwired: 8 in, 2 out]
          }
          frame "Power On-Off" {
            n143 = Format Into String(format string="%s", initial string=w236, "pause?" ("message")) -> (resulting string=w234:string)  [unwired: 1 in, 1 out]
            n144 = case shown="False" w235 {
              selector: w235 -> [w241 w252]
              tunnel: w234 -> [_ w255]
              tunnel: w233 -> [w240 w253]
              tunnel: [w239 w251] -> w230
              frame False {
                n145 = property on="M1 Enable" class="Bool (strict)"() -> ("Value"=w247:bool)  [unwired: 2 in, 2 out]
                n146 = property on="M2 Enable" class="Bool (strict)"() -> ("Value"=w246:bool)  [unwired: 2 in, 2 out]
                n147 = Not(x=w247) -> (.not. x?=w245:bool)
                n148 = Not(x=w246) -> (.not. x?=w244:bool)
                n149 = And(x=w245, y=w244) -> (x .and. y?=w242:bool)
                n150 = case shown="False" w242 {
                  tunnel: "At least one head must be \nenabled to run on" ("message") -> [_ w250]
                  tunnel: w241 -> [_ w249]
                  tunnel: [w248 w249] -> w239
                  tunnel: w240 -> [w248 _]
                  frame False {
                  }
                  frame True {
                    n151 = One Button Dialog(message=w250) -> ()  [unwired: 1 in, 1 out]
                  }
                }
              }
              frame True {
                n152 = Two Button Dialog(message=w255) -> (T button?=w254:bool)  [unwired: 2 in]
                n153 = Select(t=w253, s=w254, f=w252) -> (s? t:f=w251:bool)
              }
            }
            n154 = Unbundle By Name(w228) -> ("Network Data Down"=w227:T32, "NS Enqueuer"=w231:refnum<class "Message Enqueuer.lvclass">)
            n155 = Bundle By Name(cluster=w227, "System Power On Off"=w230, "New Data"=NS_New_Data."System Power") -> (w232:T32)
            n156 = call "Send Send Commands.vi"("Set Temp"=w232, "Message Enqueuer"=w231) -> ()  [unwired: 8 in, 2 out]
          }
          frame Default {
          }
        }
      }
      event "Config Data": Value Change {
        n157 = event-data() -> ()  [unwired: 1 in, 1 out]
        n158 = call "Send Save Config.vi"("Message Enqueuer"=w256) -> ()  [unwired: 9 in, 2 out]
      }
      event "Tuning.Login TO", "Tuning.Fixed Y-Range", "Tuning.Temp Unit", "Tuning.Average Graph": Value Change {
        n159 = event-data() -> ("CtlRef"=w263:refnum<vi>)  [unwired: 1 in]
        n160 = Unbundle By Name(w260) -> ("System Status"=w257:T33, "M1 Status"=w259:T34, "M2 Status"=w258:T34)
        n161 = property class="Ctl"(reference=w263) -> ("Label.Text"=w262:string)  [unwired: 1 in, 2 out]
        n162 = case shown="\"Temp Unit\"" w262 {
          tunnel: "Tuning" -> [w282 _ w339 _]
          tunnel: w259 -> [w268 _ _ _]
          tunnel: w258 -> [w267 _ _ _]
          tunnel: w257 -> [_ _ w336 _]
          frame "Fixed Y-Range", Default {
            n163 = Unbundle By Name(w282) -> ("Y-scale"=w266:bool, "Fixed Y-Range"=w265:dbl)
            n164 = Unbundle By Name(w268) -> ("Set Temp"=w281:dbl, "Evap Temp"=w280:dbl, "Case Temp"=w279:dbl, "TSD Temp"=w278:dbl, "Intec Feedback"=w277:dbl)
            n165 = Unbundle By Name(w267) -> ("Set Temp"=w276:dbl, "Evap Temp"=w275:dbl, "Case Temp"=w274:dbl, "TSD Temp"=w273:dbl)
            n166 = Build Array(w276, w275, w274, w273) -> (w271:dbl[])
            n167 = Build Array(w281, w280, w279, w278, w277) -> (w272:dbl[])
            n168 = control-ref of="M2 Main Waveform"() -> (w269:refnum<vi>)
            n169 = control-ref of="M1 Main Waveform"() -> (w270:refnum<vi>)
            n170 = case shown="True" w266 {
              tunnel: w270 -> [w287 w303]
              tunnel: w272 -> [_ w302]
              tunnel: w269 -> [w284 w301]
              tunnel: w271 -> [_ w300]
              tunnel: [T28."Disabled and Grayed Out" ("Disabled") T28."Enabled" ("Disabled")] -> w264
              tunnel: w265 -> [_ w288]
              frame False {
                # "Y- Autoscale"
                n171 = property on="Property Node" class="WFChart (strict)"(reference=w287, "YScale.ScaleFit"=u8 2 ("Y Scale.Scale Fit")) -> ()  [unwired: 1 in, 2 out]
                n172 = property on="Property Node" class="WFChart (strict)"(reference=w284, "YScale.ScaleFit"=u8 2 ("Y Scale.Scale Fit")) -> ()  [unwired: 1 in, 2 out]
              }
              frame True {
                # "Manually fix the Y-scale"
                n173 = Array Max & Min(array=w302) -> (max value=w296:dbl, min value=w297:dbl)  [unwired: 2 out]
                n174 = Array Max & Min(array=w300) -> (max value=w291:dbl, min value=w292:dbl)  [unwired: 2 out]
                n175 = Add(x=w296, y=w288) -> (x+y=w298:dbl)
                n176 = Subtract(x=w297, y=w288) -> (x-y=w299:dbl)
                n177 = Add(x=w291, y=w288) -> (x+y=w293:dbl)
                n178 = Subtract(x=w292, y=w288) -> (x-y=w294:dbl)
                n179 = property on="Property Node" class="WFChart (strict)"(reference=w303, "YScale.Maximum"=w298, "YScale.Minimum"=w299, "YScale.ScaleFit"=u8 0 ("Y Scale.Scale Fit")) -> ()  [unwired: 1 in, 2 out]
                n180 = property on="Property Node" class="WFChart (strict)"(reference=w301, "YScale.Maximum"=w293, "YScale.Minimum"=w294, "YScale.ScaleFit"=u8 0 ("Y Scale.Scale Fit")) -> ()  [unwired: 1 in, 2 out]
              }
            }
            n181 = property on="Fixed Y-Range" class="DigNum (strict)"("DisabledEnum"=w264) -> ()  [unwired: 2 in, 2 out]
          }
          frame "Average Graph" {
          }
          frame "Temp Unit" {
            w321 = waveform(dbl)[][] [] ("M1 Main Waveform")
            n182 = Unbundle By Name(w336) -> ("SubCooling"=w338:dbl, "SuperHeat"=w337:dbl, "Discharge Temp"=w331:dbl, "Liquid Temp"=w330:dbl, "Suction Temp"=w329:dbl, "Ambient Temp"=w328:dbl)
            n183 = Unbundle By Name(w339) -> ("Temp Unit"=w304:bool)
            n184 = property on="Manual Controls" class="Clust (strict)"("Value"=T17 {"Manual Bypass Mode"=[], "M1 Heater output"=0.0, "M1 EEV Manual"=0, "M2 Heater Output"=0.0, "M2 EEV Manual"=0} ("Manual Controls")) -> ()  [unwired: 2 in, 2 out]
            n185 = Build Array("Temperature" ("Command"), "Subcool" ("Command"), "Superheat" ("Command")) -> (w311:string[])
            n186 = Select(t="°C" ("Command"), s=w304, f="°F" ("Command")) -> (s? t:f=w310:string)
            n187 = Build Array(w338, w337, w331, w330, w329, w328) -> (w341:dbl[])
            n188 = for {
              tunnel: w310 -> [w344]
              tunnel: w311 -> [w343] mode=indexing
              tunnel: [w342] -> w312 mode=indexing
              n189 = Format Into String(format string="(%s)", initial string=w343, w344) -> (resulting string=w342:string)  [unwired: 1 in, 1 out]
            }
            n190 = for {
              tunnel: w341 -> [w354] mode=indexing
              tunnel: [w355] -> w340 mode=indexing
              tunnel: w304 -> [w356]
              n191 = expression code="5/9*(x-32)"(w354) -> (w357:dbl)
              n192 = Select(t=w357, s=w356, f=w354) -> (s? t:f=w355:dbl)
            }
            n193 = property on="M2 Main Waveform" class="WFChart (strict)"("History Data"=w321) -> ()  [unwired: 2 in, 2 out]
            n194 = property on="M1 Main Waveform" class="WFChart (strict)"("History Data"=w321) -> ()  [unwired: 2 in, 2 out]
            n195 = Index Array(array=w312) -> (element #1=w313:string, element #2=w314:string, element #3=w315:string)  [unwired: 3 in]
            n196 = property on="Ambient Temp" class="WFChart (strict)"("YScale.NameLbl.Text"=w313) -> ()  [unwired: 2 in, 2 out]
            n197 = property on="Subcool" class="Knob (strict)"("Caption.Text"=w314) -> ()  [unwired: 2 in, 2 out]
            n198 = property on="Superheat" class="Knob (strict)"("Caption.Text"=w315) -> ()  [unwired: 2 in, 2 out]
            n199 = Index Array(array=w340) -> (element #1=w333:dbl, element #2=w332:dbl, element #3=w325:dbl, element #4=w324:dbl, element #5=w323:dbl, element #6=w322:dbl)  [unwired: 6 in]
            n200 = control-ref of="M1 Graphs"() -> (w319:refnum<vi>)
            n201 = control-ref of="M2 Graphs"() -> (w318:refnum<vi>)
            n202 = control-ref of="System Graphs"() -> (w317:refnum<vi>)
            n203 = Build Array(w319, w318, w317) -> (w316:refnum<vi>[])
            n204 = Bundle By Name(cluster=T6 {"Ambient Temp"=77.534379824996, "Suction Temp"=77.78750485181808, "Condensor Temp"=77.29531729966402, "Discharge Temp"=78.09687988460064, "Bypass Steps"=72.0} ("System Graphs"), "Discharge Temp"=w325, "Condensor Temp"=w324, "Suction Temp"=w323, "Ambient Temp"=w322) -> (w326:T6)
            n205 = for {
              tunnel: w316 -> [w349] mode=indexing
              n206 = property class="Clust (strict)"(reference=w349) -> ("Controls[]"=w347:refnum<vi>[])  [unwired: 1 in, 2 out]
              n207 = for {
                tunnel: dbl[] [] ("History Data") -> [w353]
                tunnel: w347 -> [w352] mode=indexing
                tunnel: refnum<vi> refnum ("M1 Heater Power (%)") -> [w350]
                n208 = To More Specific Class(target class=w350, reference=w352) -> (specific class reference=w351:refnum<vi>)  [unwired: 1 in, 1 out]
                n209 = property class="WFChart (strict)"(reference=w351, "History Data"=w353) -> ()  [unwired: 1 in, 2 out]
              }
            }
            n210 = property on="System Graphs" class="Clust (strict)"("Value"=w326) -> ()  [unwired: 2 in, 2 out]
            n211 = Bundle By Name(cluster=T7 {"Condensing Pressure(psi)"=165.57116807812622, "Compression Ratio"=1.0119646390563775, "Subcool"=-0.3368072880168427, "Superheat"=1.4200558413526494, "Current(A)"=0.2333286882987343, "Suction Pressure(psi)"=163.4397897916897} ("Gauges"), "Subcool"=w333, "Superheat"=w332) -> (w335:T7)
            n212 = property on="Gauges" class="Clust (strict)"("Value"=w335) -> ()  [unwired: 2 in, 2 out]
          }
          frame "Login TO" {
          }
        }
      }
      event "Cascade Compressor controls", "Manual Controls.Manual Bypass Mode", "Manual Controls.M1 Heater output", "Manual Controls.M1 EEV Manual", "Manual Controls.M2 Heater Output", "Manual Controls.M2 EEV Manual": Value Change {
        n213 = event-data() -> ("CtlRef"=w366:refnum<vi>, "NewVal"=w364:variant)  [unwired: 1 in]
        n214 = Unbundle By Name(w359) -> ("IP Address"=w358:string)
        n215 = property on="M1 TSD" class="Bool (strict)" props=["Value"]() -> ()  [unwired: 2 in, 3 out]
        n216 = property on="M2 TSD" class="Bool (strict)" props=["Value"]() -> ()  [unwired: 2 in, 3 out]
        n217 = property class="Ctl"(reference=w366) -> ("Caption.Text"=w365:string)  [unwired: 1 in, 2 out]
        n218 = Concatenate Strings("ni.var.psp://", w358, "/Network Shared Variables/") -> (w361:string)
        n219 = case shown="\"M2 EEV Manual\"" w365 {
          selector: w365 -> [_ w367 _ _ w396 w411 w426 w441 w452]
          tunnel: w364 -> [_ w369 w378 w386 w400 w415 w430 w445 w456]
          tunnel: w361 -> [_ w368 w380 w388 w401 w416 w431 w446 w457]
          tunnel: "Manual Controls" -> [_ _ _ _ w392 w407 w423 w437 _]
          frame Default {
          }
          frame "Cascade Compressor controls" {
            n220 = Variant To Data(type=T16 {"High Stage manual speed control"=FALSE, "Manual High stage frequency"=0.0, "Low Stage manual speed control"=FALSE, "Manual Low Stage frequency"=0.0} ("Cascade Compressor controls"), Variant=w369) -> (data=w372:T16, error out=w371:errorcluster)  [unwired: 1 in]
            n221 = Format Into String(format string="%s", initial string=w368, w367) -> (resulting string=w373:string)  [unwired: 1 in, 1 out]
            n222 = shared-variable-write(w373, w371, w372) -> ()  [unwired: 2 out]
          }
          frame "M1 TSD" {
            n223 = Variant To Data(type=FALSE ("TSD Feedback"), Variant=w378) -> (data=w376:bool, error out=w377:errorcluster)  [unwired: 1 in]
            n224 = Format Into String(format string="%s", initial string=w380, "TSD Feedback" ("input 1")) -> (resulting string=w375:string)  [unwired: 1 in, 1 out]
            n225 = shared-variable-write(w375, w377, w376) -> ()  [unwired: 2 out]
          }
          frame "M2 TSD" {
            n226 = Variant To Data(type=FALSE ("TSD Feedback"), Variant=w386) -> (data=w384:bool, error out=w385:errorcluster)  [unwired: 1 in]
            n227 = Format Into String(format string="%s", initial string=w388, "M2 TSD Feedback" ("input 1")) -> (resulting string=w383:string)  [unwired: 1 in, 1 out]
            n228 = shared-variable-write(w383, w385, w384) -> ()  [unwired: 2 out]
          }
          frame "M1 EEV Manual" {
            n229 = Unbundle By Name(w392) -> ("Manual Bypass Mode"=w394:bool[])
            n230 = Variant To Data(type=i16 0 ("M2 EEV Manual control"), Variant=w400) -> (data=w398:i16, error out=w399:errorcluster)  [unwired: 1 in]
            n231 = Format Into String(format string="%s", initial string=w401, w396) -> (resulting string=w397:string)  [unwired: 1 in, 1 out]
            n232 = Index Array(array=w394, index=1) -> (element=w391:bool)
            n233 = case shown="False" w391 {
              tunnel: w399 -> [_ w405]
              tunnel: w398 -> [_ w404]
              tunnel: w397 -> [_ w403]
              frame False {
              }
              frame True {
                n234 = shared-variable-write(w403, w405, w404) -> ()  [unwired: 2 out]
              }
            }
          }
          frame "M2 EEV Manual" {
            n235 = Unbundle By Name(w407) -> ("Manual Bypass Mode"=w409:bool[])
            n236 = Variant To Data(type=i16 0 ("M2 EEV Manual control"), Variant=w415) -> (data=w413:i16, error out=w414:errorcluster)  [unwired: 1 in]
            n237 = Format Into String(format string="%s", initial string=w416, w411) -> (resulting string=w412:string)  [unwired: 1 in, 1 out]
            n238 = Index Array(array=w409, index=3) -> (element=w406:bool)
            n239 = case shown="True" w406 {
              tunnel: w414 -> [_ w420]
              tunnel: w413 -> [_ w419]
              tunnel: w412 -> [_ w418]
              frame False {
              }
              frame True {
                n240 = shared-variable-write(w418, w420, w419) -> ()  [unwired: 2 out]
              }
            }
          }
          frame "M1 Heater output" {
            n241 = Unbundle By Name(w423) -> ("Manual Bypass Mode"=w422:bool[])
            n242 = Variant To Data(type=0.0 ("M1 Heater PWM"), Variant=w430) -> (data=w428:dbl, error out=w429:errorcluster)  [unwired: 1 in]
            n243 = Index Array(array=w422, index=0) -> (element=w421:bool)
            n244 = Format Into String(format string="%s", initial string=w431, w426) -> (resulting string=w427:string)  [unwired: 1 in, 1 out]
            n245 = case shown="False" w421 {
              tunnel: w429 -> [_ w435]
              tunnel: w428 -> [_ w434]
              tunnel: w427 -> [_ w433]
              frame False {
              }
              frame True {
                n246 = shared-variable-write(w433, w435, w434) -> ()  [unwired: 2 out]
              }
            }
          }
          frame "M2 Heater Output" {
            n247 = Unbundle By Name(w437) -> ("Manual Bypass Mode"=w439:bool[])
            n248 = Variant To Data(type=0.0 ("M1 Heater PWM"), Variant=w445) -> (data=w443:dbl, error out=w444:errorcluster)  [unwired: 1 in]
            n249 = Format Into String(format string="%s", initial string=w446, w441) -> (resulting string=w442:string)  [unwired: 1 in, 1 out]
            n250 = Index Array(array=w439, index=2) -> (element=w436:bool)
            n251 = case shown="True" w436 {
              tunnel: w444 -> [_ w450]
              tunnel: w443 -> [_ w449]
              tunnel: w442 -> [_ w448]
              frame False {
              }
              frame True {
                n252 = shared-variable-write(w448, w450, w449) -> ()  [unwired: 2 out]
              }
            }
          }
          frame "Manual Bypass Mode" {
            n253 = Variant To Data(type=bool[] [] ("Manual Bypass Mode"), Variant=w456) -> (data=w454:bool[], error out=w455:errorcluster)  [unwired: 1 in]
            n254 = Format Into String(format string="%s", initial string=w457, w452) -> (resulting string=w453:string)  [unwired: 1 in, 1 out]
            n255 = shared-variable-write(w453, w455, w454) -> ()  [unwired: 2 out]
          }
        }
      }
      event Value Change {
        n256 = event-data() -> ("NewVal"=w477:T14)  [unwired: 1 in]
        n257 = case shown="True" w477 {
          tunnel: [T29."Operator" ("Level") w497] -> w476
          frame False {
          }
          frame True {
            n258 = call "Login.vi"() -> ("OK?"=w499:bool, "Level"=w498:T29)  [unwired: 8 in, 1 out]
            n259 = case shown="True" w499 {
              tunnel: w498 -> [_ w502]
              tunnel: [T29."Operator" ("Level") w502] -> w497
              frame False {
                n260 = property on="Login" class="Bool (strict)"("Value"=T14 FALSE ("Login")) -> ()  [unwired: 2 in, 2 out]
              }
              frame True {
              }
            }
          }
        }
        n261 = case shown="\"Guest\"" w476 {
          tunnel: [i32[] [0, 1, 2, 3, 4, 5] ("Page array") i32[] [0, 1, 2, 3] ("Page array") i32[] [0, 1, 2] ("Page array") i32[] [0, 1, 2] ("Page array")] -> w474
          tunnel: [TRUE ("Visible") TRUE ("Visible") FALSE ("Visible") FALSE ("Visible")] -> w465
          tunnel: [T28."Enabled" ("Disabled") T28."Enabled" ("Disabled") T28."Disabled and Grayed Out" ("Disabled") T28."Disabled and Grayed Out" ("Disabled")] -> w467
          frame "Supervisor" {
          }
          frame "Engineer" {
          }
          frame "Operator", Default {
          }
          frame "Guest" {
          }
        }
        n262 = control-ref of="Tab Control"() -> (w475:refnum<vi>)
        n263 = property on="Manual Controls" class="Clust (strict)"("DisabledEnum"=w467) -> ()  [unwired: 2 in, 2 out]
        n264 = property class="TabCtl (strict)"(reference=w475) -> ("Pages"=w473:refnum<vi>[])  [unwired: 1 in, 2 out]
        n265 = Array Size(array=w474) -> (size(s)=w472:i32)
        n266 = property on="Reboot RT" class="Bool"("Visible"=w465) -> ()  [unwired: 2 in, 2 out]
        n267 = property on="Config Data" class="Bool"("Visible"=w465) -> ()  [unwired: 2 in, 2 out]
        n268 = property on="Subcool" class="Knob (strict)"("Visible"=w465) -> ()  [unwired: 2 in, 2 out]
        n269 = property on="Superheat" class="Knob (strict)"("Visible"=w465) -> ()  [unwired: 2 in, 2 out]
        n270 = Split 1D Array(array=w473, index=w472) -> (first subarray=w469:refnum<vi>[], second subarray=w468:refnum<vi>[])
        n271 = control-ref of="?"() -> (w464:refnum<vi>)
        n272 = control-ref of="?"() -> (w463:refnum<vi>)
        n273 = control-ref of="?"() -> (w462:refnum<vi>)
        n274 = control-ref of="?"() -> (w461:refnum<vi>)
        n275 = control-ref of="?"() -> (w460:refnum<vi>)
        n276 = control-ref of="?"() -> (w459:refnum<vi>)
        n277 = Build Array(w464, w463, w462, w461, w460, w459) -> (w466:refnum<vi>[])
        n278 = for {
          tunnel: w468 -> [w480] mode=indexing
          tunnel: T25."Page Disabled & Grayed" ("Page Enabled State") -> [w481]
          n279 = property class="Page"(reference=w480, "PageEnb"=w481) -> ()  [unwired: 1 in, 2 out]
        }
        n280 = for {
          tunnel: w465 -> [w479]
          tunnel: w466 -> [w478] mode=indexing
          n281 = property class="DigNum (strict)"(reference=w478, "Visible"=w479) -> ()  [unwired: 1 in, 2 out]
        }
        n282 = for {
          tunnel: w469 -> [w482] mode=indexing
          tunnel: T25."Page Enabled" ("Page Enabled State") -> [w483]
          n283 = property class="Page"(reference=w482, "PageEnb"=w483) -> ()  [unwired: 1 in, 2 out]
        }
      }
      event "Datalog": Value Change {
        n284 = event-data() -> ()  [unwired: 1 in, 1 out]
        n285 = disable-structure shown="Enabled" {
          disable-tunnel: w503 -> [_ w534]
          frame Enabled {
            n286 = local read "IP Address"() -> (w504:string)
            n287 = Format Into String(format string="%s/files", initial string="http://" ("host uri prefix"), w504) -> (resulting string=w519:string)  [unwired: 1 in, 1 out]
            n288 = call "WebDAV FGV.vi"("WebDAV States"=WebDAV_states."Open Sess", "host uri prefix"=w519) -> ("error out"=w512:errorcluster)  [unwired: 7 in, 2 out]
            n289 = call "WebDAV FGV.vi"("WebDAV States"=WebDAV_states."Refresh Dir", "error in (no error)"=w512, "relative uri"="/u/") -> ("error out"=w505:errorcluster, "file list"=w516:T35[])  [unwired: 6 in, 1 out]
            n290 = Reverse 1D Array(array=w516) -> (reversed array=w517:T35[])
            n291 = for {
              tunnel: w517 -> [w526] mode=indexing
              tunnel: [w521] -> w513 mode=indexing if=w520
              tunnel: [w524] -> w514 mode=indexing if=w520
              tunnel: [w522] -> w515 mode=indexing if=w520
              n292 = Unbundle By Name(w526) -> ("display name"=w521:string, "size"=w525:u64, "last modification"=w523:timestamp)
              n293 = String To Path(string=w521) -> (path=w529:path)
              n294 = Format Date/Time String(seconds (now)=w523) -> (date/time string=w522:string)  [unwired: 2 in]
              n295 = call <vilib>:"Get File Extension.vi"("file"=w529) -> ("lowercase file extension"=w528:string)  [unwired: 6 in, 4 out]
              n296 = Number To Decimal String(number=w525) -> (decimal integer string=w524:string)  [unwired: 1 in]
              n297 = Equal?(x=w528, y="tdms") -> (x = y?=w520:bool)
            }
            n298 = Build Array(w513, w514, w515) -> (w518:string[][])
            n299 = Transpose 2D Array(2D array=w518) -> (transposed array=w506:string[][])
            n300 = call "Dialog TDMS Datalog.vi"("Error In"=w505, "Logdata"=w506) -> ()  [unwired: 9 in, 1 out]
          }
          frame Disabled {
            n301 = Unbundle By Name(w534) -> ("Connected System"=w536:refnum<vi>)
            n302 = property class="Str"(reference=w536) -> ("Value"=w533:string)  [unwired: 1 in, 2 out]
            n303 = Unbundle By Name(w534) -> ("NS Enqueuer"=w531:refnum<class "Message Enqueuer.lvclass">)
            n304 = call "Send Close Connection.vi"("Message Enqueuer"=w531) -> ("Message Enqueuer out"=w530:refnum<class "Message Enqueuer.lvclass">)  [unwired: 9 in, 1 out]
            n305 = xnode ("Match Regular Expression")("input string"=w533, "regular expression"="\\b[0-9]+\\.[0-9]+\\.[0-9]+\\.[0-9]+") -> ("whole match"=w532:string)  [unwired: 4 in, 4 out]
            n306 = call "Send Open Connection.vi"("IP"=w532, "Message Enqueuer"=w530) -> ()  [unwired: 8 in, 2 out]
          }
        }
      }
    }
  }
  n307 = call-parent "Actor Core.vi"("error in"=w22, "Panel Actor in"=w16) -> ("error out"=w14:errorcluster, "Actor out"=w15:refnum<class "Actor.lvclass">)  [unwired: 8 in]
  n308 = flat-sequence {
    tunnel: w20 -> [w653]
    tunnel: w15 -> [w652]
    tunnel: w14 -> [w651]
    frame #0 {
      n309 = invoke class="VI" method="FP.Close"() -> ()  [unwired: 3 in, 3 out]
      n310 = Unregister For Events(event registration refnum=w653) -> ()  [unwired: 1 in, 1 out]
      "error out" <- w651
      "Actor out" <- w652
    }
  }
